vi "WHD_VEten_0.1.3._WS_BIDIR_Calibr.vi"() -> ()   [LabVIEW 2015]
uses:
  <vilib>/LabVIEW Targets/FPGA/cRIO/shared/nicrio_ModuleControls/nicrio_cRIO-9234_DataRatesRing2.ctl
  <vilib>/RTwatchdog.llb/Watchdog expiration actions.ctl
  <vilib>/userDefined/High Color/nirio_resource_hc.ctl
  <vilib>/FPGAPlugInAG/cRIO-9031/niLvFpga_Open_cRIO-9031.vi
  <vilib>/Utility/error.llb/Error Cluster From Error Code.vi
  <vilib>/rvi/errors/niLvFpgaAdjustHostInterfaceError.vi
  <vilib>/Utility/file.llb/Write Delimited Spreadsheet (string).vi
  <vilib>/FPGAPlugInAG/cRIO-9031/niLvFpga_Run_cRIO-9031.vi
  <vilib>/rvi/interface/common/niFpgaWaitOnOcc.vi
  <vilib>/FPGAPlugInAG/cRIO-9031/niLvFpga_Reset_cRIO-9031.vi
  <vilib>/Utility/config.llb/Write Key (Double).vi
  <vilib>/FPGAPlugInAG/cRIO-9031/niLvFpga_Close_cRIO-9031.vi
  <vilib>/rvi/interface/nirviOpenFPGA/nirviOpenFPGA.xnode
  FPGA Bitfiles/W&RDArabia_FPGATarget_FPGA8a2wsBIdirec_yJvL9yuTbZw.lvbitx
  <vilib>/rvi/interface/nirviReadWriteControl/nirviReadWriteControl.xnode
  <vilib>/rvi/interface/nirviMethod/nirviMethod.xnode
  <vilib>/rvi/interface/nirviCloseFPGA/nirviCloseFPGA.xnode
  <vilib>/NI_Real-Time Target Support.lvlib
  <vilib>/rvi/errors/niLvFpgaMergeErrorWithErrorCode.vi
  AURA_Wheel/Json2Labv.lvlib
  AURA_Wheel/AuraWheelAPI/AuraWheel.lvlib
  NiFpgaLv.dll
  <vilib>/FPGAPlugInAG/cRIO-9031/niLvFpga_ConfigureFifo_cRIO-9031.vi
  <vilib>/FPGAPlugInAG/cRIO-9031/niLvFpga_StartFifo_cRIO-9031.vi
  <vilib>/FPGAPlugInAG/cRIO-9031/niLvFpga_ReadFifo_cRIO-9031.vi
  <vilib>/FPGAPlugInAG/cRIO-9031/niLvFpga_StopFifo_cRIO-9031.vi
  <vilib>/Utility/config.llb/NI_LVConfig.lvlib
panel:
  in  "Developer commad":string
  out "Save calibration":bool
  out "calibration log":path
  out "Pattern amplitude (g)":dbl=1.02
  out "Pattern frequency (Hz)":dbl=159.2
  out "Folder":path
  out "Report":string
  out "path calib":path
  out "AURA wheel test":bool
  out "LOG.txt":path
  out "Report_AURA":string
  out "RFID_Error":errorcluster
  out "error FPGA":errorcluster
  out "error AURA":errorcluster
  out "error manipulacion archivos":errorcluster
  out "Response headers":string
  out "Max RMS Ruedas":dbl[][](array[numeric])
  out "TAGs LR6":string[](array[string])
  out "TAGs HEX":string[](array[string])
  out "Parar":bool
  out "result":bool
  out "TAGs":string[](array[string])
  out "Temperatura (ºC)":dbl
  out "V (m/s)":dbl
  out "Digital?":bool=TRUE
  out "Watchdog config":T1={"reset"=FALSE, "occurrence"=FALSE, "trigger protocol"=enum."active high", "trigger line"=enum."none", "disable watchdog on VI exit"=TRUE}
  out "Tiempo de adquisicion":dbl=10.0
  out "Adquirir":bool
  out "Nº Ruedas 1":i32
  out "NºRuedas 2":i32
  out "Disco Duro Disponible (bytes)":i64
  out "Buffer Overflow":bool
  out "Buffer Underflow":bool
  out "Archivo\nvalido?":bool
  out "Número de ejes detectados":i32
  out "Ejes_convoy":i32
  out "Tiempo de paso (s)":dbl
  out "created path":path
  out "Nombre de archivo":path[](array[path])
  out "LR6 IP address":string="192.168.106.94"
  out "Port LR6":u16=2001
  out "T fuera rango":bool
  out "Frecuencia de muestreo (Hz)":dbl=25600.0
  out "Escaneos de la FIFO por canal":u32=5000
  out "Tiempo extra al detector de paso (s)":dbl=1.0
  out "dt RMS":dbl=256.0
  out "Frecuencia de muestreo y módulo CRIO":T2=2 items=["51.200 kS/s (NI 9234)"=1, "25.600 kS/s (NI 9234)"=2, "17.067 kS/s (NI 9234)"=3, "12.800 kS/s (NI 9234)"=4, "10.240 kS/s (NI 9234)"=5, "8.533 kS/s (NI 9234)"=6, "7.314 kS/s (NI 9234)"=7, "6.400 kS/s (NI 9234)"=8, "5.689 kS/s (NI 9234)"=9, "5.120 kS/s (NI 9234)"=10, "4.654 kS/s (NI 9234)"=11, "4.267 kS/s (NI 9234)"=12, "3.938 kS/s (NI 9234)"=13, "3.657 kS/s (NI 9234)"=14, "3.413 kS/s (NI 9234)"=15, "3.200 kS/s (NI 9234)"=16, "3.012 kS/s (NI 9234)"=17, "2.845 kS/s (NI 9234)"=18, "2.695 kS/s (NI 9234)"=19, "2.560 kS/s (NI 9234)"=20, "2.438 kS/s (NI 9234)"=21, "2.328 kS/s (NI 9234)"=22, "2.226 kS/s (NI 9234)"=23, "2.133 kS/s (NI 9234)"=24, "2.048 kS/s (NI 9234)"=25, "1.969 kS/s (NI 9234)"=26, "1.896 kS/s (NI 9234)"=27, "1.829 kS/s (NI 9234)"=28, "1.765 kS/s (NI 9234)"=29, "1.707 kS/s (NI 9234)"=30, "1.652 kS/s (NI 9234)"=31]
  out "Puerto RFID":u16=2189
  out "IP RFID":string="192.168.106.99"
  out "Offset_rueda WS 2":fxp<+/-,24,-4>=0.004999998956918716 format="%.27g"
  out "Count(mSec)":u32=2
  out "RFID NEM on?":bool
  out "RFID LR6 on?":bool
  out "Canal cero WS1?":bool
  out "Canal cero WS2":bool
  out "Inicio pasada 2":timestamp
  in  "Calibration":bool
  out "Direccion 0?":bool
  out "Boton Adquirir?":bool
  out "RuedaDetectada2?":bool=TRUE
  out "RuedaDetectada1?":bool=TRUE
  out "Timeout ruedas":dbl
  out "Borrar archivos\nadquisicion con error":bool
  out "Able watchdog?":bool
  out "Reset watchdog?":bool
  out "Leer config RFID NEM":bool
  out "bytes to read":i32
  out "DeviceAddress":u8
  out "timeout ms (60000)":i32
  out "Max archivos":u32=2
  out "Bytes libre despues de borrar":u32=2
  out "Bytes min libre":u32=2
  out "Nº de acelerómetros":i32
  out "Nº inductivos":i32
  out "Offset_rueda WS 1":fxp<+/-,24,-4>=0.004999998956918716 format="%.27g"
  out "TAGs_AURAwheel":string[][](array[string])
  out "Plataformas?":bool
  out "Nº Ejes":i32[](array[numeric])
  out "Nº UTs":i32
  out "it-read-LR6":i32[](array[numeric])
  out "it-LR6":i32
  out "RFID_LR6_Error":errorcluster
  out "Series_flota":string[](array[string])
  out "Tabla_flota":string[][](array[string])
  out "Puntos medios de las ventanas":dbl[][](array[numeric])
  out "configuration file path":path=path "c:/Parametros.cfg"
  out "IP synchr":string
  out "data":cluster{"status":string}
  out "confRFID":path=path "c:/RFID/TAGS.csv"
  out "TAGS leidos":path=path "c:/RFID/TAGS.csv"
  out "Use Aura?":bool
  out "Parametros AuraWheel":string[](array[string])
  out "Parámetros acelerómetros":dbl[](array[numeric])
  out "Fin":bool
  out "Contador":i32=1
  out "Path LOG":path=path "c:/TEST"
  out "Fallo fotocelula":bool
  out "Path_Borrar":path=path "c:/Trenes"
  out "Longitud de la unidad":dbl
  out "Aviso no detección":string
  out "Time to Acquire Block (ms)":i32
  out "Distancia de acelerómetros":dbl[](array[numeric])
  out "Block Size":u32
  out "Distancias generales":dbl[](array[numeric])
  out "Reset del controlador":bool
  out "Parar la aplicación":bool
  out "date/time string":string
  out "Timeout ruedas":bool
  out "Tiempo":dbl
  out "Inicio pasada":timestamp
  out "Ultimo TEST":timestamp
  out "Fuente":bool=TRUE
  out "RFID_ID":refnum<k5>
  out "DC OK":string
  out "Aviso temperatura":string
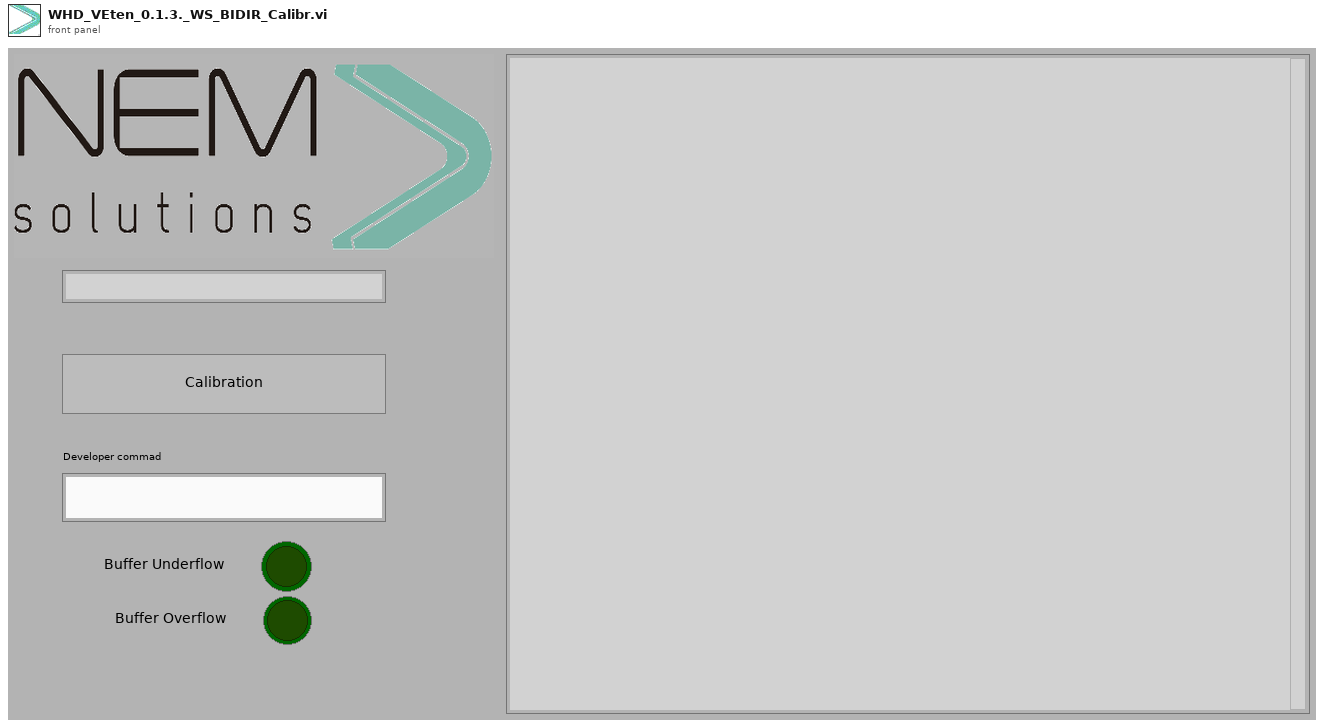
[diagram p1: front panel]
types:
  T1 = typedef "Watchdog expiration actions.ctl" = cluster{"reset":bool, "occurrence":bool, "trigger protocol":enum16{"active high", "active low", "open collector"}, "trigger line":enum16{"none", "line 0", "line 1", "line 2", "line 3", "line 4", "line 5", "line 6", "line 7", "SMB line 0"}, "disable watchdog on VI exit":bool}
  T2 = typedef "nicrio_cRIO-9234_DataRatesRing2.ctl" = u8
  T3 = typedef "nirio_resource_hc.ctl" = tag
  T4 = enum16{"Standard", "Buffered", "CRLF", "Immediate"}
  T5 = enum16{"open", "replace", "create", "open or create", "replace or create", "replace or create with confirmation"}
  T6 = enum16{"big-endian, network order", "native, host order", "little-endian"}
  T7 = cluster{"error IO":errorcluster, bool[], u32[], string[], dbl[]}
  T8 = cluster{"error out":errorcluster, dbl[], "TAGs":string[], "Direccion 0?":bool}
  T9 = cluster{"g_ts":dbl, "p_sp":dbl, "p_tp":dbl, "p_tg":cluster{"tg_n":dbl, "tg_t":string}[], "p_ax":cluster{"ax_n":dbl, "ax_sp":dbl, "ax_wh":cluster{"wh_p":dbl, "wh_a1":dbl, "wh_a2":dbl, "wh_a3":dbl, "wh_a4":dbl}[]}[]}
  T10 = cluster{"Frecuencia de muestreo y módulo CRIO":T2, "Count(mSec)":u32, "Frecuencia de muestreo (Hz)":dbl, "Escaneos de la FIFO por canal":u32, "Nº inductivos":i32, "Nº de acelerómetros":i32}
  T11 = typedef "NI_LVConfig.lvlib/Config Data RefNum.ctl" = refnum<k1>
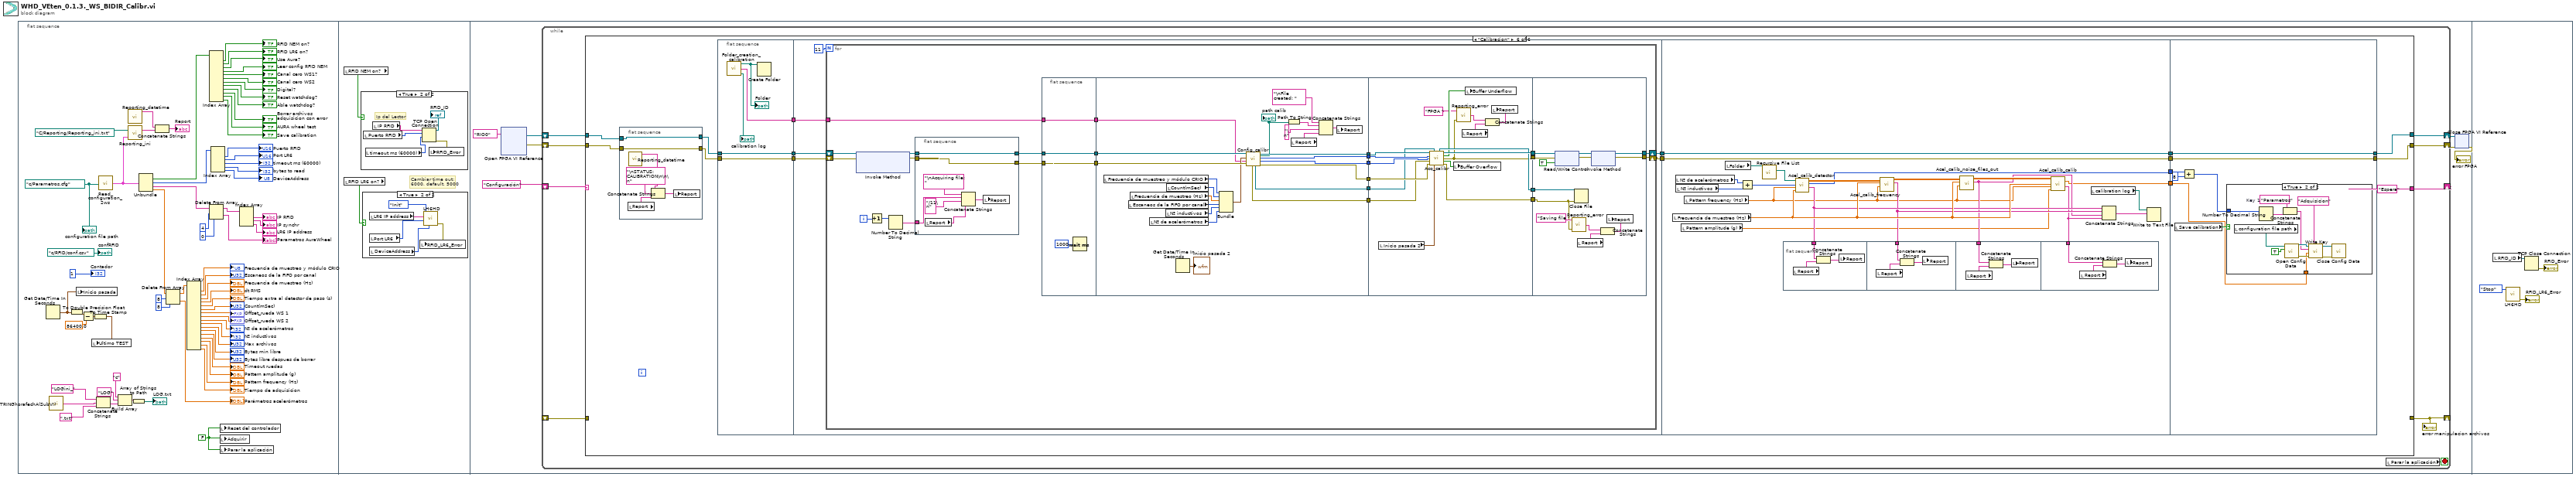
[diagram p0: block diagram]
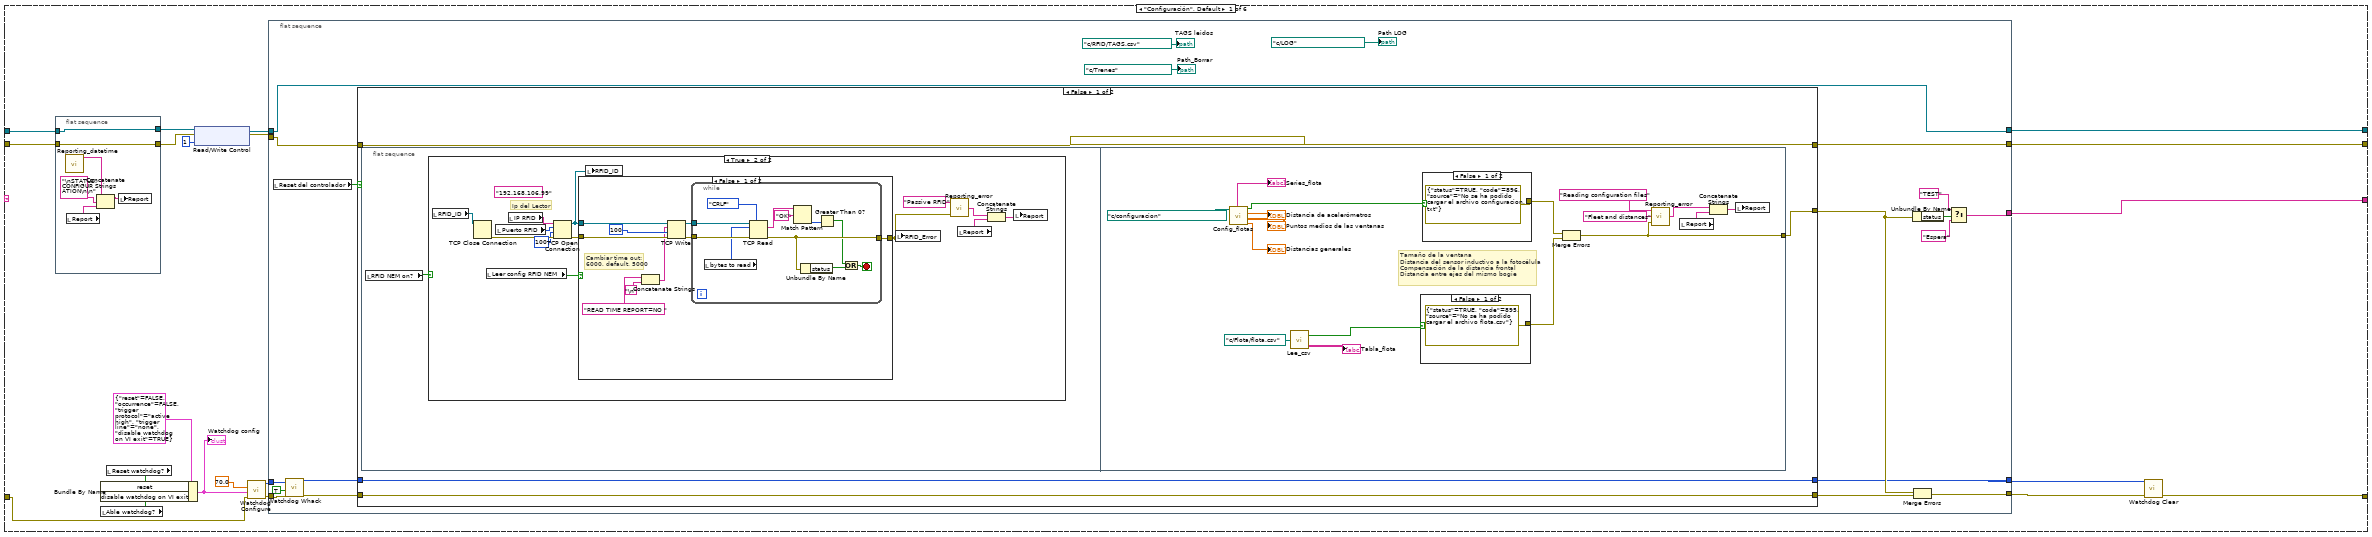
[diagram p4: hidden frame]
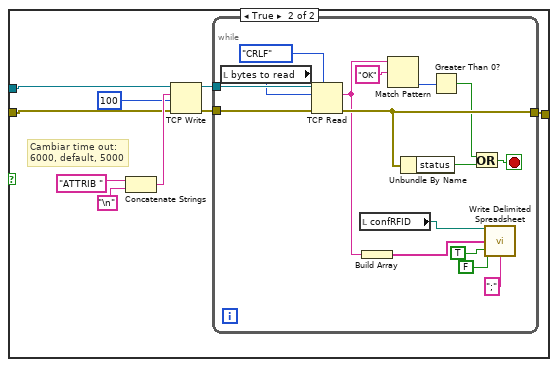
[diagram p6: hidden frame]
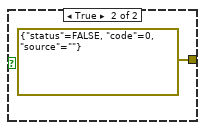
[diagram p7: hidden frame]
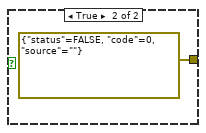
[diagram p8: hidden frame]
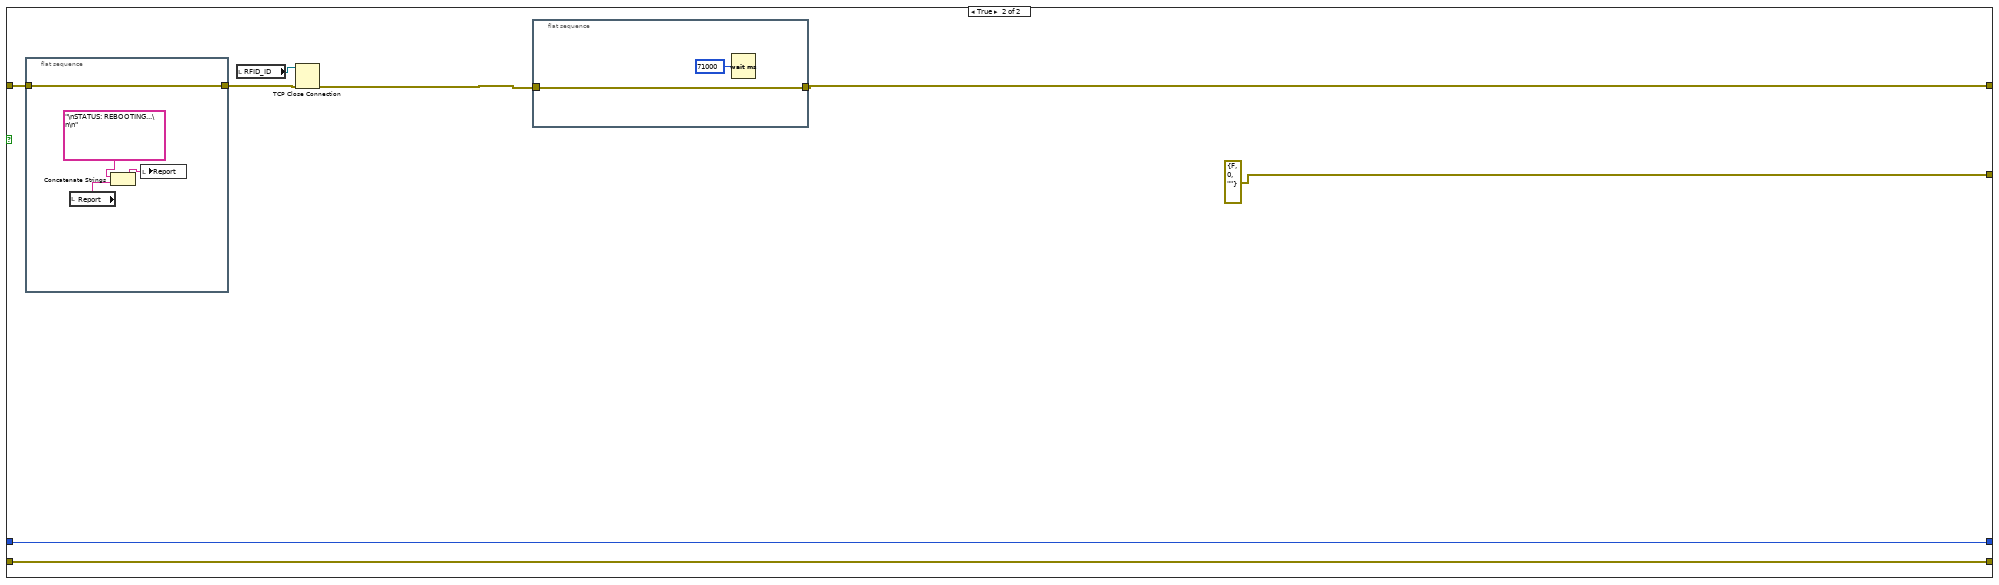
[diagram p9: hidden frame]
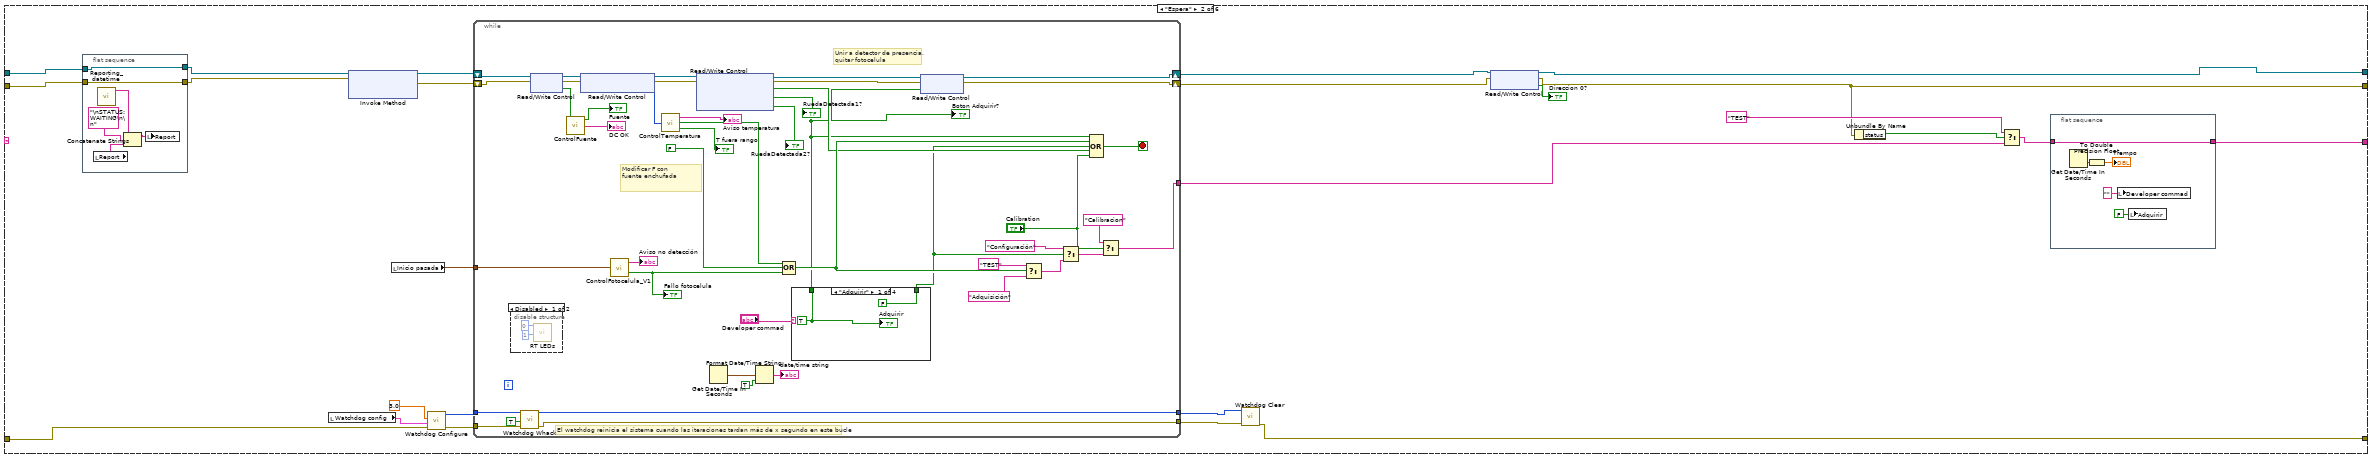
[diagram p10: hidden frame]
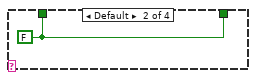
[diagram p11: hidden frame]
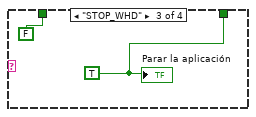
[diagram p12: hidden frame]
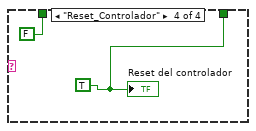
[diagram p13: hidden frame]
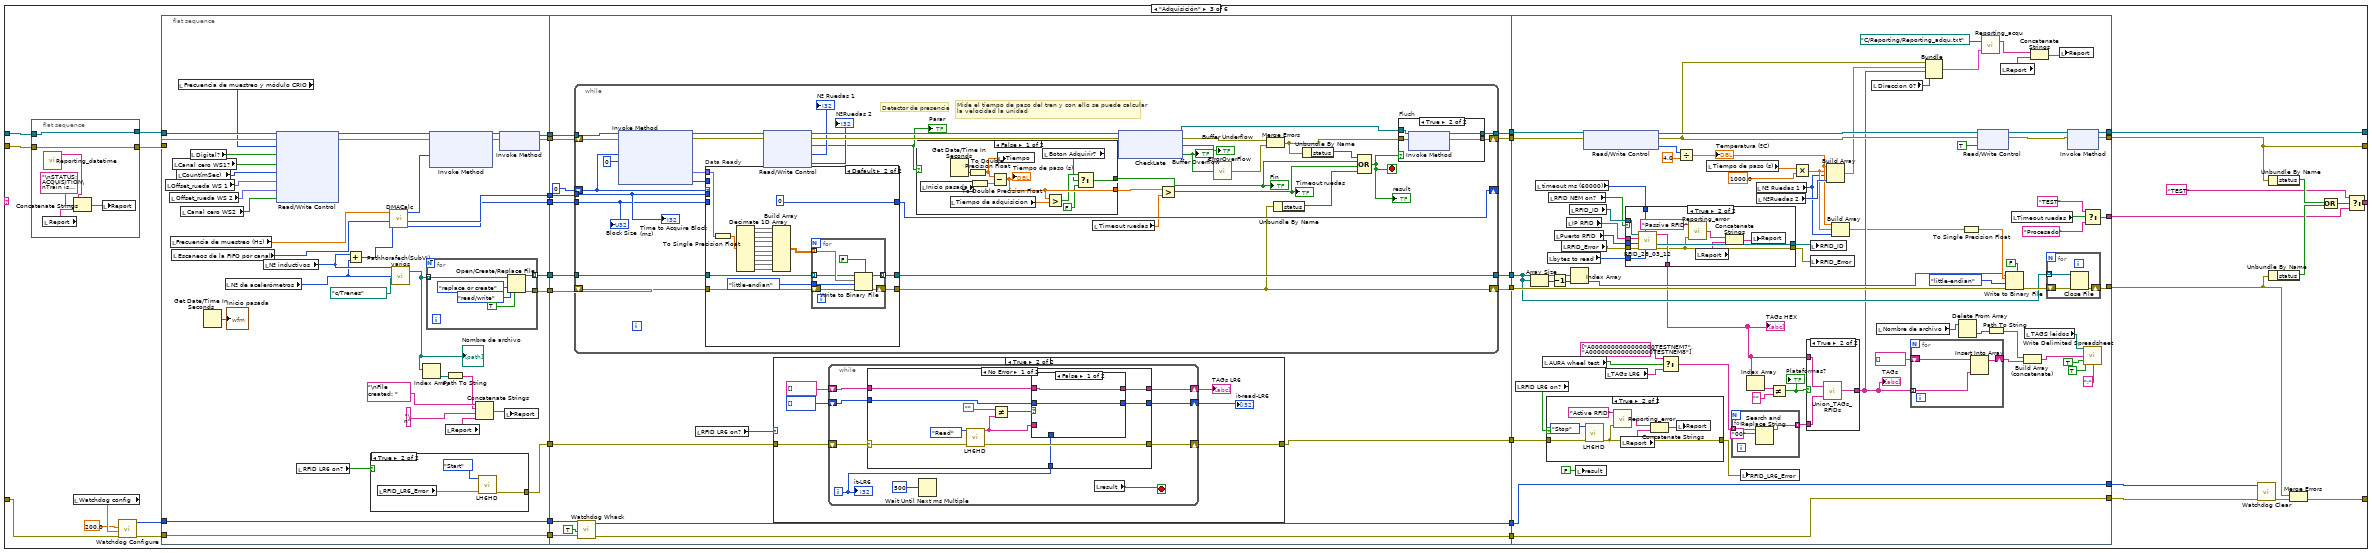
[diagram p15: hidden frame]
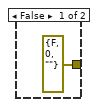
[diagram p16: hidden frame]
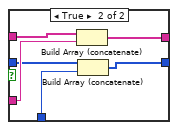
[diagram p18: hidden frame]
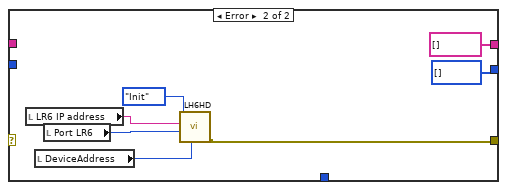
[diagram p19: hidden frame]
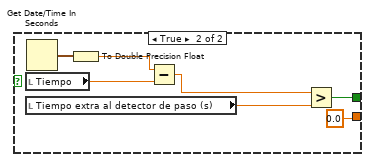
[diagram p20: hidden frame]
diagram:
  n1 = flat-sequence {
    frame #0 {
      w1 = FALSE ("Reset del controlador")
      w63 = path "c:/Parametros.cfg" ("configuration file path")
      n2 = Get Date/Time In Seconds() -> (seconds since 1Jan1904=w68:timestamp)
      n3 = call "STRINGhorafechA(SubVI).vi"() -> ("STRINGhora_fecha"=w12:string)
      n4 = To Double Precision Float(number=w68) -> (double precision float=w70:dbl)
      n5 = local write "Inicio pasada"(w68) -> ()
      n6 = Subtract(x=w70, y=86400.0) -> (x-y=w69:dbl)
      n7 = To Time Stamp(1:w69) -> (0:w67:timestamp)
      n8 = local write "Ultimo TEST"(w67) -> ()
      n9 = Concatenate Strings("LOGini_" ("string"), w12, ".txt" ("string")) -> (w14:string)
      n10 = call "Read_configuration_2ws.vi"("configuration file path"=w63) -> ("output cluster"=w18:T7)
      n11 = Build Array("c", "LOG" ("element"), w14) -> (w11:string[])
      n12 = call "Reporting_ini.vi"("Configuration cluster"=w18, "address repoting"=path "C:/Reporting/Reporting_ini.txt" ("file (use dialog)")) -> ("Reporting"=w17:string)  [unwired: 1 in]
      n13 = call "Reporting_datetime.vi"() -> ("String"=w15:string)  [unwired: 11 in]
      n14 = Array of Strings to Path(0:w11) -> (2:→"LOG.txt":path)  [unwired: 1 out]
      n15 = Unbundle(w18) -> (w66:bool[], w65:u32[], w58:string[], w62:dbl[])  [unwired: 1 out]
      n16 = Concatenate Strings(w15, w17) -> (→"Report":string)
      n17 = Delete From Array(array=w62, length=8, index=8) -> (deleted portion=→"Parámetros acelerómetros":dbl[], array with subset deleted=w61:dbl[])
      n18 = Index Array(array=w61) -> (element #1=→"Frecuencia de muestreo y módulo CRIO":dbl, element #2=→"Escaneos de la FIFO por canal":dbl, element #3=→"Frecuencia de muestreo (Hz)":dbl, element #4=→"dt RMS":dbl, element #5=→"Tiempo extra al detector de paso (s)":dbl, element #6=→"Count(mSec)":dbl, element #7=→"Offset_rueda WS 1":dbl, element #8=→"Offset_rueda WS 2":dbl, element #9=→"Nº de acelerómetros":dbl, element #10=→"Nº inductivos":dbl, element #11=→"Max archivos":dbl, element #12=→"Bytes min libre":dbl, element #13=→"Bytes libre despues de borrar":dbl, element #14=→"Timeout ruedas":dbl, element #15=→"Pattern amplitude (g)":dbl, element #16=→"Pattern frequency (Hz)":dbl, element #17=→"Tiempo de adquisicion":dbl)  [unwired: 17 in]
      n19 = Index Array(array=w66) -> (element #1=→"RFID NEM on?":bool, element #2=→"RFID LR6 on?":bool, element #3=→"Use Aura?":bool, element #4=→"Leer config RFID NEM":bool, element #5=→"Canal cero WS1?":bool, element #6=→"Canal cero WS2":bool, element #7=→"Digital?":bool, element #8=→"Reset watchdog?":bool, element #9=→"Able watchdog?":bool, element #10=→"Borrar archivos\nadquisicion con error":bool, element #11=→"AURA wheel test":bool, element #12=→"Save calibration":bool)  [unwired: 12 in]
      n20 = Delete From Array(array=w58, length=4, index=0) -> (deleted portion=→"Parametros AuraWheel":string[], array with subset deleted=w57:string[])
      n21 = Index Array(array=w65) -> (element #1=→"Puerto RFID":u32, element #2=→"Port LR6":u32, element #3=→"timeout ms (60000)":u32, element #4=→"bytes to read":u32, element #5=→"DeviceAddress":u32)  [unwired: 5 in]
      n22 = local write "Reset del controlador"(w1) -> ()
      n23 = local write "Adquirir"(w1) -> ()
      n24 = local write "Parar la aplicación"(w1) -> ()
      n25 = Index Array(array=w57) -> (element #1=→"IP RFID":string, element #2=→"IP synchr":string, element #3=→"LR6 IP address":string)  [unwired: 3 in]
      "Contador" <- 1
      "confRFID" <- path "c:/RFID/conf.csv" ("file path (use dialog)")
      "configuration file path" <- w63
    }
    frame #1 {
      # "Cambiar time out:\n6000, default, 5000"
      n26 = local read "RFID NEM on?"() -> (w73:bool)
      n27 = local read "RFID LR6 on?"() -> (w72:bool)
      n28 = case shown="True" w73 {
        frame False {
        }
        frame True {
          # "Ip del Lector"
          n29 = local read "Puerto RFID"() -> (w81:u16)
          n30 = local read "timeout ms (60000)"() -> (w79:i32)
          n31 = local read "IP RFID"() -> (w82:string)
          n32 = TCP Open Connection(address=w82, remote port or service name=w81, timeout ms (60000)=w79) -> (connection ID=→"RFID_ID":refnum<k5>, error out=w80:errorcluster)  [unwired: 1 in, 1 out]
          n33 = local write "RFID_Error"(w80) -> ()
        }
      }
      n34 = case shown="True" w72 {
        frame False {
        }
        frame True {
          n35 = local read "LR6 IP address"() -> (w74:string)
          n36 = local read "Port LR6"() -> (w75:u16)
          n37 = local read "DeviceAddress"() -> (w76:u8)
          n38 = call "LH6HD.vi"("DeviceAddress"=w76, "Reader Port"=w75, "IP Address"=w74, "Action"=enum16{"Init", "Start", "Read", "Stop", "Exit"}."Init") -> ("error out"=w78:errorcluster)  [unwired: 6 in, 1 out]
          n39 = local write "RFID_LR6_Error"(w78) -> ()
        }
      }
    }
    frame #2 {
      n40 = xnode "Open FPGA VI Reference"("resource name"=T3 "RIO0") -> ("FPGA VI Reference Out"=w90:refnum<k20>, "error out"=w89:errorcluster)  [unwired: 1 in]
      n41 = while {
        shift-right: [w91] -> _
        shift-left: "Configuración" -> [w99]
        shift-right: [w93] -> w86
        shift-left: w90 -> [w98]
        shift-right: [w92] -> w85
        shift-left: w89 -> [w97]
        shift-right: [w96] -> _
        shift-left: _ -> [w95]
        stop <- w94 stop-if-true
        n42 = case shown="\"Calibracion\"" w99 {
          tunnel: [w109 w262 w352 w709 w957 "Espera"] -> w91
          tunnel: [w119 w250 w366 w698 w956 w1030] -> w93
          tunnel: [w120 w249 w367 w696 w955 w1029] -> w92
          tunnel: w98 -> [w103 w248 w338 w699 w956 w1035]
          tunnel: w97 -> [w102 w247 w337 w697 w948 w1034]
          tunnel: [w116 w256 w364 w694 w947 _] -> w96
          tunnel: w95 -> [w108 w261 w348 w708 w944 _]
          frame "Configuración", Default {
            n43 = flat-sequence {
              tunnel: w103 -> [w126]
              tunnel: w102 -> [w125]
              tunnel: [w126] -> w101
              tunnel: [w125] -> w100
              frame #0 {
                n44 = call "Reporting_datetime.vi"() -> ("String"=w121:string)  [unwired: 11 in]
                n45 = local read "Report"() -> (w122:string)
                n46 = Concatenate Strings(w121, "\nSTATUS: CONFIGURATION\n\n", w122) -> (w124:string)
                n47 = local write "Report"(w124) -> ()
              }
            }
            n48 = local read "Able watchdog?"() -> (w113:bool)
            n49 = local read "Reset watchdog?"() -> (w114:bool)
            n50 = Bundle By Name(cluster=T1 {"reset"=FALSE, "occurrence"=FALSE, "trigger protocol"=enum."active high", "trigger line"=enum."none", "disable watchdog on VI exit"=TRUE} ("expiration actions"), "reset"=w114, "disable watchdog on VI exit"=w113) -> (w107:T1)
            "Watchdog config" <- w107
            n51 = xnode "Read/Write Control"("FPGA VI Reference In"=w101, "error in"=w100, "Cycles to Filter"=u16 1) -> ("FPGA VI Reference Out"=w112:refnum<k20>, "error out"=w111:errorcluster)
            n52 = call <vilib>:"Watchdog Configure.vi"("error in (no error)"=w108, "expiration actions"=w107, "timeout (1 sec)"=70.0) -> ("error out"=w104:errorcluster, "watchdogID"=w105:u64)  [unwired: 1 in, 2 out]
            n53 = flat-sequence {
              tunnel: [w137] -> w120
              tunnel: [w145] -> w109
              tunnel: w112 -> [w138]
              tunnel: [w138] -> w119
              tunnel: [w140] -> w117
              tunnel: w111 -> [w135]
              tunnel: [w132] -> w118
              tunnel: w105 -> [w128]
              tunnel: w104 -> [w127]
              frame #0 {
                n54 = local read "Reset del controlador"() -> (w134:bool)
                n55 = call <vilib>:"Watchdog Whack.vi"("error in (no error)"=w127, "reset watchdog after expire? (F)"=TRUE, "watchdogID in"=w128) -> ("error out"=w130:errorcluster, "watchdogID out"=w131:u64)  [unwired: 2 in, 1 out]
                n56 = case shown="False" w134 {
                  tunnel: w135 -> [w150 w233]
                  tunnel: [w150 w236] -> w137
                  tunnel: [w147 errorcluster {"status"=FALSE, "code"=0, "source"=""} ("error IO")] -> w136
                  tunnel: [w149 w235] -> w132
                  tunnel: w131 -> [w149 w235]
                  tunnel: w130 -> [w148 w234]
                  tunnel: [w148 w234] -> w129
                  frame False {
                    n57 = flat-sequence {
                      tunnel: [w210] -> w147
                      frame #0 {
                        n58 = local read "RFID NEM on?"() -> (w151:bool)
                        n59 = case shown="True" w151 {
                          frame False {
                          }
                          frame True {
                            (unwired) "192.168.106.99" ("address")
                            # "Ip del Lector"
                            n60 = local read "RFID_ID"() -> (w163:refnum<k5>)
                            n61 = TCP Close Connection(connection ID=w163) -> (error out=w164:errorcluster)  [unwired: 2 in, 1 out]
                            n62 = local read "Leer config RFID NEM"() -> (w157:bool)
                            n63 = local read "Puerto RFID"() -> (w161:u16)
                            n64 = local read "IP RFID"() -> (w160:string)
                            n65 = TCP Open Connection(address=w160, remote port or service name=w161, timeout ms (60000)=100, error in (no error)=w164) -> (connection ID=w162:refnum<k5>, error out=w158:errorcluster)  [unwired: 1 out]
                            n66 = case shown="False" w157 {
                              tunnel: w162 -> [w173 w187]
                              tunnel: [w171 w185] -> w156
                              tunnel: w158 -> [w168 w186]
                              frame False {
                                # "Cambiar time out:\n6000, default, 5000"
                                n67 = Concatenate Strings("READ TIME REPORT=NO " ("data in"), "\n") -> (w165:string)
                                n68 = TCP Write(connection ID=w173, data in=w165, error in (no error)=w168, 9:100 ("timeout ms (25000)")) -> (connection ID out=w169:refnum<k5>, error out=w170:errorcluster)  [unwired: 1 out]
                                n69 = while {
                                tunnel: w170 -> [w183]
                                tunnel: w169 -> [w182]
                                tunnel: [w181] -> w171
                                stop <- w178 stop-if-true
                                n70 = local read "bytes to read"() -> (w174:i32)
                                n71 = TCP Read(connection ID=w182, bytes to read=w174, error in (no error)=w183, 7:T4."CRLF" ("mode (standard)")) -> (data out=w176:string, error out=w181:errorcluster)  [unwired: 1 in, 1 out]
                                n72 = Match Pattern(string=w176, regular expression="OK") -> (offset past match=w179:i32)  [unwired: 4 out]
                                n73 = Unbundle By Name(w181) -> ("status"=w177:bool)
                                n74 = Greater Than 0?(x=w179) -> (x > 0?=w175:bool)
                                n75 = Or(x=w175, y=w177) -> (x .or. y?=w178:bool)
                                }
                              }
                              frame True {
                                # "Cambiar time out:\n6000, default, 5000"
                                n76 = Concatenate Strings("ATTRIB " ("data in"), "\n") -> (w193:string)
                                n77 = TCP Write(connection ID=w187, data in=w193, error in (no error)=w186, 9:100 ("timeout ms (25000)")) -> (connection ID out=w190:refnum<k5>, error out=w189:errorcluster)  [unwired: 1 out]
                                n78 = while {
                                tunnel: w189 -> [w208]
                                tunnel: w190 -> [w207]
                                tunnel: [w206] -> w185
                                stop <- w203 stop-if-true
                                n79 = local read "bytes to read"() -> (w194:i32)
                                n80 = TCP Read(connection ID=w207, bytes to read=w194, error in (no error)=w208, 7:T4."CRLF" ("mode (standard)")) -> (data out=w197:string, error out=w206:errorcluster)  [unwired: 1 in, 1 out]
                                n81 = local read "confRFID"() -> (w196:path)
                                n82 = Build Array(w197) -> (w195:string[])
                                n83 = Match Pattern(string=w197, regular expression="OK") -> (offset past match=w204:i32)  [unwired: 4 out]
                                n84 = Unbundle By Name(w206) -> ("status"=w202:bool)
                                n85 = Greater Than 0?(x=w204) -> (x > 0?=w201:bool)
                                n86 = Or(x=w201, y=w202) -> (x .or. y?=w203:bool)
                                n87 = call-poly <vilib>:"Write Delimited Spreadsheet.vi"("file path (dialog if empty)"=w196, "1D data"=w195, "append to file? (F)"=FALSE ("transpose? (no:F)"), "transpose? (F)"=TRUE ("append to file? (new file:F)"), "delimiter (\\t)"=";" ("delimiter (\\t)")) -> ()  [unwired: 9 in, 2 out]
                                }
                              }
                            }
                            n88 = local write "RFID_ID"(w162) -> ()
                            n89 = local write "RFID_Error"(w156) -> ()
                            n90 = call "Reporting_error.vi"("error out 2"=w156, "Concept"="Passive RFID") -> ("Reporting"=w153:string)  [unwired: 1 in]
                            n91 = local read "Report"() -> (w154:string)
                            n92 = Concatenate Strings(w153, w154) -> (w152:string)
                            n93 = local write "Report"(w152) -> ()
                          }
                        }
                      }
                      frame #1 {
                        # "Tamaño de la ventana\nDistancia del sensor inductivo a la fotocélula\nCompensación de la distancia frontal\nDistancia entre ejes del mismo bogie"
                        n94 = call "Config_flotas.vi"("file path (dialog if empty)"=path "c:/configuracion") -> ("Distancias generales"=→"Distancias generales":dbl[], "Puntos medios de las ventanas"=→"Puntos medios de las ventanas":dbl[][], "Distancia de acelerómetros"=→"Distancia de acelerómetros":dbl[], "Distacias y medidas de dispositivos"=w223:bool, "Series_flota"=→"Series_flota":string[])  [unwired: 3 in]
                        n95 = call "Lee_csv.vi"("Path"=path "c:/Flota/flota.csv") -> ("Tabla_flota"=→"Tabla_flota":string[][], "Lectura_OK?"=w220:bool)
                        n96 = case shown="False" w220 {
                          tunnel: [errorcluster {"status"=TRUE, "code"=895, "source"="No se ha podido cargar el archivo flota.csv"} ("error out") errorcluster {"status"=FALSE, "code"=0, "source"=""} ("error out")] -> w224
                          frame False {
                          }
                          frame True {
                          }
                        }
                        n97 = case shown="False" w223 {
                          tunnel: [errorcluster {"status"=TRUE, "code"=896, "source"="No se ha podido cargar el archivo configuracion.txt"} ("error out") errorcluster {"status"=FALSE, "code"=0, "source"=""} ("error out")] -> w225
                          frame False {
                          }
                          frame True {
                          }
                        }
                        n98 = Merge Errors(w225, w224) -> (w210:errorcluster)
                        n99 = call "Reporting_error.vi"("error out 2"=w210, "Concept explanation"="Fleet and distances", "Concept"="Reading configuration files") -> ("Reporting"=w212:string)
                        n100 = local read "Report"() -> (w211:string)
                        n101 = Concatenate Strings(w212, w211) -> (w213:string)
                        n102 = local write "Report"(w213) -> ()
                      }
                    }
                  }
                  frame True {
                    n103 = flat-sequence {
                      tunnel: w233 -> [w242]
                      tunnel: [w242] -> w232
                      frame #0 {
                        n104 = local read "Report"() -> (w241:string)
                        n105 = Concatenate Strings("\nSTATUS: REBOOTING...\n\n", w241) -> (w239:string)
                        n106 = local write "Report"(w239) -> ()
                      }
                    }
                    n107 = local read "RFID_ID"() -> (w238:refnum<k5>)
                    n108 = TCP Close Connection(connection ID=w238, error in (no error)=w232) -> (error out=w231:errorcluster)  [unwired: 2 out]
                    n109 = flat-sequence {
                      tunnel: [w244] -> w236
                      tunnel: w231 -> [w244]
                      frame #0 {
                        n110 = Wait (ms)(milliseconds to wait=u32 71000) -> ()  [unwired: 1 out]
                      }
                    }
                  }
                }
                n111 = Unbundle By Name(w136) -> ("status"=w146:bool)
                n112 = Merge Errors(w136, w129) -> (w140:errorcluster)
                n113 = Select(t="TEST", s=w146, f="Espera") -> (s? t:f=w145:string)
                "Path_Borrar" <- path "c:/Trenes" ("file path (use dialog)")
                "Path LOG" <- path "c:/LOG" ("file path (use dialog)")
                "TAGS leidos" <- path "c:/RFID/TAGS.csv" ("file path (use dialog)")
              }
            }
            n114 = call <vilib>:"Watchdog Clear.vi"("error in (no error)"=w117, "watchdogID in"=w118) -> ("error out"=w116:errorcluster)  [unwired: 5 in]
          }
          frame "Espera" {
            n115 = flat-sequence {
              tunnel: w248 -> [w275]
              tunnel: w247 -> [w274]
              tunnel: [w275] -> w246
              tunnel: [w274] -> w245
              frame #0 {
                n116 = local read "Report"() -> (w271:string)
                n117 = call "Reporting_datetime.vi"() -> ("String"=w270:string)  [unwired: 11 in]
                n118 = Concatenate Strings(w270, "\nSTATUS: WAITING\n\n", w271) -> (w273:string)
                n119 = local write "Report"(w273) -> ()
              }
            }
            n120 = local read "Watchdog config"() -> (w255:T1)
            n121 = xnode "Invoke Method"("FPGA VI Reference In"=w246, "error in"=w245) -> ("FPGA VI Reference Out"=w265:refnum<k20>, "error out"=w264:errorcluster)  [unwired: 1 in]
            n122 = local read "Inicio pasada"() -> (w269:timestamp)
            n123 = call <vilib>:"Watchdog Configure.vi"("error in (no error)"=w261, "expiration actions"=w255, "timeout (1 sec)"=3.0) -> ("error out"=w260:errorcluster, "watchdogID"=w259:u64)  [unwired: 1 in, 2 out]
            n124 = while {
              tunnel: [w286] -> w268
              shift-right: [w295] -> w251
              shift-left: w265 -> [w305]
              shift-right: [w294] -> w252
              shift-left: w264 -> [w304]
              tunnel: w269 -> [w308]
              tunnel: w260 -> [w292]
              tunnel: w259 -> [w293]
              tunnel: [w291] -> w258
              tunnel: [w290] -> w257
              stop <- w284 stop-if-true
              # "Modificar F con\nfuente enchufada"
              # "Unir a detector de presencia,\nquitar fotocelula"
              # "El watchdog reinicia el sistema cuando las iteraciones tardan más de x segundo en este bucle"
              n125 = disable-structure shown="Disabled" {
                frame Disabled {
                  n126 = call <vilib>:"RT LEDs.vi"("State"=1, "LED Num"=0) -> ()  [unwired: 1 in, 5 out]
                }
                frame Enabled {
                }
              }
              n127 = call <vilib>:"Watchdog Whack.vi"("error in (no error)"=w292, "reset watchdog after expire? (F)"=TRUE, "watchdogID in"=w293) -> ("error out"=w290:errorcluster, "watchdogID out"=w291:u64)  [unwired: 2 in, 1 out]
              n128 = xnode "Read/Write Control"("FPGA VI Reference In"=w305, "error in"=w304) -> ("FPGA VI Reference Out"=w317:refnum<k20>, "error out"=w316:errorcluster, "DC OK"=w321:bool)
              n129 = call "ControlFuente.vi"("DC OK 3"=w321) -> ("DC OK 2"=→"Fuente":bool, "DC OK"=→"DC OK":string)  [unwired: 1 out]
              n130 = xnode "Read/Write Control"("FPGA VI Reference In"=w317, "error in"=w316) -> ("FPGA VI Reference Out"=w312:refnum<k20>, "error out"=w311:errorcluster, "Chassis Temperature"=w319:i16)
              n131 = call "ControlFotocelula_V1.vi"("Tiempo de entrada a espera"=w308) -> ("Aviso no detección"=→"Aviso no detección":string, "Boolean"=w309:bool)
              "Fallo fotocelula" <- w309
              n132 = call "ControlTemperatura.vi"("Chassis Temperature"=w319) -> ("Aviso temperatura"=→"Aviso temperatura":string, "Boolean"=w313:bool, "T fuera rango"=→"T fuera rango":bool)
              n133 = xnode "Read/Write Control"("FPGA VI Reference In"=w312, "error in"=w311) -> ("FPGA VI Reference Out"=w307:refnum<k20>, "error out"=w306:errorcluster, "Detector de presencia"=w300:bool, "RuedaDetectada1?"=→"RuedaDetectada1?":bool, "RuedaDetectada2?"=→"RuedaDetectada2?":bool)
              n134 = Get Date/Time In Seconds() -> (seconds since 1Jan1904=w302:timestamp)
              n135 = Format Date/Time String(seconds (now)=w302, UTC format=TRUE) -> (date/time string=→"date/time string":string)  [unwired: 1 in]
              n136 = Compound Arithmetic op=OR(w313, FALSE ("value"), w309) -> (w310:bool)
              n137 = case shown="\"Adquirir\"" "Developer commad" {
                tunnel: [w327 w328 FALSE ("Adquirir") FALSE ("Adquirir")] -> w283
                tunnel: [FALSE ("Adquirir") w328 w329 w331] -> w282
                frame "Adquirir" {
                  w327 = TRUE ("Adquirir")
                  "Adquirir" <- w327
                }
                frame Default {
                  w328 = FALSE ("Adquirir")
                }
                frame "STOP_WHD" {
                  w329 = TRUE ("Adquirir")
                  "Parar la aplicación" <- w329
                }
                frame "Reset_Controlador" {
                  w331 = TRUE ("Adquirir")
                  "Reset del controlador" <- w331
                }
              }
              "Boton Adquirir?" <- w283
              n138 = xnode "Read/Write Control"("FPGA VI Reference In"=w307, "error in"=w306, "Fotocélula"=w283) -> ("FPGA VI Reference Out"=w295:refnum<k20>, "error out"=w294:errorcluster)
              n139 = Select(t="TEST", s=w310, f="Adquisición") -> (s? t:f=w322:string)
              n140 = Select(t="Configuración", s=w282, f=w322) -> (s? t:f=w288:string)
              n141 = Compound Arithmetic op=OR(w283, w310, w282, w300, "Calibration") -> (w284:bool)
              n142 = Select(t="Calibracion", s="Calibration", f=w288) -> (s? t:f=w286:string)
            }
            n143 = call <vilib>:"Watchdog Clear.vi"("error in (no error)"=w257, "watchdogID in"=w258) -> ("error out"=w256:errorcluster)  [unwired: 5 in]
            n144 = xnode "Read/Write Control"("FPGA VI Reference In"=w251, "error in"=w252) -> ("FPGA VI Reference Out"=w250:refnum<k20>, "error out"=w249:errorcluster, "Direccion 0?"=→"Direccion 0?":bool)
            n145 = Unbundle By Name(w249) -> ("status"=w267:bool)
            n146 = Select(t="TEST", s=w267, f=w268) -> (s? t:f=w263:string)
            n147 = flat-sequence {
              tunnel: [w279] -> w262
              tunnel: w263 -> [w279]
              frame #0 {
                n148 = Get Date/Time In Seconds() -> (seconds since 1Jan1904=w280:timestamp)
                n149 = To Double Precision Float(number=w280) -> (double precision float=→"Tiempo":dbl)
                n150 = local write "Developer commad"("" ("Developer commad")) -> ()
                n151 = local write "Adquirir"(FALSE ("Adquirir")) -> ()
              }
            }
          }
          frame "Adquisición" {
            n152 = flat-sequence {
              tunnel: w338 -> [w378]
              tunnel: w337 -> [w377]
              tunnel: [w378] -> w336
              tunnel: [w377] -> w335
              frame #0 {
                n153 = local read "Report"() -> (w374:string)
                n154 = call "Reporting_datetime.vi"() -> ("String"=w373:string)  [unwired: 11 in]
                n155 = Concatenate Strings(w373, "\nSTATUS: ACQUISITION\nTrain is passing\n\n", w374) -> (w376:string)
                n156 = local write "Report"(w376) -> ()
              }
            }
            n157 = local read "Watchdog config"() -> (w349:T1)
            n158 = call <vilib>:"Watchdog Configure.vi"("error in (no error)"=w348, "expiration actions"=w349, "timeout (1 sec)"=200.0) -> ("error out"=w346:errorcluster, "watchdogID"=w347:u64)  [unwired: 1 in, 2 out]
            n159 = flat-sequence {
              tunnel: w335 -> [w412]
              tunnel: w336 -> [w413]
              tunnel: [w411] -> w363
              tunnel: [w410] -> w362
              tunnel: [w409] -> w361
              tunnel: [w408] -> w360
              tunnel: [w407] -> w359
              tunnel: [w406] -> w358
              tunnel: [w396] -> w351
              tunnel: w347 -> [w395]
              tunnel: w346 -> [w394]
              tunnel: [w395] -> w345
              tunnel: [w394] -> w344
              tunnel: [w428] -> w372
              tunnel: [w445] -> w371
              tunnel: [w444] -> w370
              tunnel: [w443] -> w369
              tunnel: [w436] -> w368
              tunnel: w363 -> [w442]
              tunnel: w362 -> [w441]
              tunnel: w361 -> [w440]
              tunnel: w360 -> [w439]
              tunnel: w359 -> [w438]
              tunnel: w358 -> [w437]
              tunnel: w351 -> [w434]
              tunnel: [w433] -> w350
              tunnel: w345 -> [w432]
              tunnel: w344 -> [w431]
              tunnel: [w429] -> w343
              tunnel: w372 -> [w609]
              tunnel: w371 -> [w604]
              tunnel: w370 -> [w603]
              tunnel: w369 -> [w623]
              tunnel: [w650] -> w355
              tunnel: w368 -> [w652]
              tunnel: [w639] -> w365
              tunnel: [w640] -> w367
              tunnel: [w641] -> w366
              tunnel: w350 -> [w618]
              tunnel: w343 -> [w610]
              tunnel: [w610] -> w341
              tunnel: [w609] -> w340
              frame #0 {
                n160 = local read "Offset_rueda WS 1"() -> (w389:fxp<+/-,24,-4>)
                n161 = local read "Offset_rueda WS 2"() -> (w390:fxp<+/-,24,-4>)
                n162 = local read "Frecuencia de muestreo (Hz)"() -> (w404:dbl)
                n163 = local read "Escaneos de la FIFO por canal"() -> (w393:u32)
                n164 = local read "Canal cero WS1?"() -> (w398:bool)
                n165 = local read "Count(mSec)"() -> (w397:u32)
                n166 = local read "Frecuencia de muestreo y módulo CRIO"() -> (w400:T2)
                n167 = local read "Canal cero WS2"() -> (w388:bool)
                n168 = local read "Digital?"() -> (w399:bool)
                n169 = Get Date/Time In Seconds() -> (seconds since 1Jan1904=→"Inicio pasada":timestamp)
                n170 = local read "Nº de acelerómetros"() -> (w386:i32)
                n171 = local read "Nº inductivos"() -> (w387:i32)
                n172 = xnode "Read/Write Control"("FPGA VI Reference In"=w413, "error in"=w412, "Data Rate"=w400, "Digital?"=w399, "Canal cero WS1?"=w398, "Count(mSec)"=w397, "Offset_WS1"=w389, "Offset_WS2"=w390, "Canal cero WS2?"=w388) -> ("FPGA VI Reference Out"=w403:refnum<k20>, "error out"=w402:errorcluster)
                n173 = local read "RFID LR6 on?"() -> (w391:bool)
                n174 = Add(x=w387, y=w386) -> (x+y=w392:i32)
                n175 = case shown="True" w391 {
                  tunnel: [errorcluster {"status"=FALSE, "code"=0, "source"=""} ("error out") w418] -> w396
                  frame False {
                  }
                  frame True {
                    n176 = local read "RFID_LR6_Error"() -> (w419:errorcluster)
                    n177 = call "LH6HD.vi"("error in (no error)"=w419, "Action"=enum16{"Init", "Start", "Read", "Stop", "Exit"}."Start") -> ("error out"=w418:errorcluster)  [unwired: 8 in, 1 out]
                  }
                }
                n178 = call "DMACalc.vi"("Number of Channels"=w392, "Number of Samples"=w393, "Rate (Hz)"=w404) -> ("Block Size"=w408:u32, "Time to Acquire Block (ms)"=w409:i32, "Host Buffer Size"=w414:u32)  [unwired: 6 in]
                n179 = call "Pathhorafech(SubVI)_varios.vi"("Folder path"=path "c:/Trenes", "Nº de acelerómetros"=w386, "Nº inductivos"=w387) -> ("Acel_Paths"=w382:path[])  [unwired: 1 in, 1 out]
                "Nombre de archivo" <- w382
                n180 = Index Array(array=w382) -> (element=w381:path)  [unwired: 1 in]
                n181 = for {
                  tunnel: w382 -> [w423] mode=indexing
                  tunnel: [w422] -> w407 mode=indexing
                  tunnel: [w421] -> w406
                  n182 = Open/Create/Replace File(file path (use dialog)=w423, operation (0:open)=T5."replace or create", access (0:read/write)=enum16{"read/write", "read-only", "write-only"}."read/write", disable buffering (F)=TRUE) -> (refnum out=w422:refnum<file>, error out=w421:errorcluster)  [unwired: 1 in, 2 out]
                }
                n183 = xnode "Invoke Method"("FPGA VI Reference In"=w403, "error in"=w402, "Requested Depth"=w414) -> ("FPGA VI Reference Out"=w416:refnum<k20>, "error out"=w415:errorcluster)  [unwired: 1 out]
                n184 = local read "Report"() -> (w385:string)
                n185 = Path To String(path=w381) -> (string=w379:string)
                n186 = Concatenate Strings("\nFile created: ", w379, "\n", w385) -> (w384:string)
                n187 = xnode "Invoke Method"("FPGA VI Reference In"=w416, "error in"=w415) -> ("FPGA VI Reference Out"=w411:refnum<k20>, "error out"=w410:errorcluster)
                n188 = local write "Report"(w384) -> ()
              }
              frame #1 {
                n189 = while "Data Acquisition" {
                  tunnel: w442 -> [w496]
                  shift-right: [w520] -> _
                  shift-left: u32 0 ("t") -> [w516]
                  tunnel: w440 -> [w521]
                  tunnel: w439 -> [w519]
                  shift-right: [w522] -> w444
                  shift-left: w441 -> [w513]
                  tunnel: [w517] -> w445
                  tunnel: w438 -> [w500]
                  tunnel: [w501] -> w443
                  shift-right: [w499] -> w436
                  shift-left: w437 -> [w509]
                  stop <- w518 stop-if-true
                  # "Detector de presencia"
                  # "Mide el tiempo de paso del tren y con ello se puede calcular\nla velocidad la unidad"
                  n190 = xnode "Invoke Method"("FPGA VI Reference In"=w496, "error in"=w513, "Number of Elements"=w516, "Timeout (ms)"=0) -> ("FPGA VI Reference Out"=w493:refnum<k20>, "error out"=w498:errorcluster, "Data"=w512:fxp<+/-,24,4>[], "Elements Remaining"=w514:u32)
                  n191 = case "Data Ready" shown="Default" w516 {
                    tunnel: w521 -> [w544 _]
                    tunnel: [w543 u32 0 ("t")] -> w520
                    tunnel: w519 -> [w545 _]
                    tunnel: w514 -> [w542 _]
                    tunnel: w512 -> [_ w567]
                    tunnel: w509 -> [w541 w566]
                    tunnel: [w541 w568] -> w499
                    tunnel: w500 -> [w540 w565]
                    tunnel: [w540 w564] -> w501
                    frame 0 {
                      # "En este caso se compara los elementos que quedan\nen la FIFO del controlador con el tamaño dell bloque\nque aparece en el panel frontal. Si el número de \nelementos en la FIFO es mayor o igual que el tamaño\n del bloque se pasa al siguiente caso y se guardan \nlos datos en un archivo. El reloj que aparece es una\nespera para no consumir recursos."
                      n192 = Greater Or Equal?(x=w542, y=w545) -> (x >= y?=w546:bool)
                      n193 = case shown="False" w546 {
                        tunnel: [u32 0 ("Block Size") w550] -> w543
                        tunnel: [w549 0 ("t")] -> w547
                        tunnel: w544 -> [w549 _]
                        tunnel: w545 -> [_ w550]
                        frame False {
                        }
                        frame True {
                        }
                      }
                      n194 = call "WaitMinTimeBetweenCall.vi"("Minimum ms between calls"=w547) -> ()  [unwired: 2 in]
                    }
                    frame Default {
                      n195 = To Single Precision Float(number=w567) -> (single precision float=w554:sgl[])
                      n196 = Decimate 1D Array(w554) -> (w560:sgl[], w563:sgl[], w562:sgl[], w561:sgl[], w559:sgl[], w558:sgl[], w557:sgl[], w556:sgl[], w555:sgl[], w552:sgl[])
                      n197 = Build Array(w560, w563, w562, w561, w559, w558, w557, w556, w555, w552) -> (w553:sgl[][])
                      n198 = for {
                        tunnel: T6."little-endian" ("byte order (0:big-endian, network order)") -> [w577]
                        shift-right: [w571] -> w568
                        shift-left: w566 -> [w572]
                        tunnel: w553 -> [w575] mode=indexing
                        tunnel: w565 -> [w574] mode=indexing
                        tunnel: [w573] -> w564 mode=indexing
                        n199 = Write to Binary File(file (use dialog)=w574, data=w575, error in=w572, 5:FALSE ("prepend array or string size? (T)"), 9:w577) -> (refnum out=w573:refnum<file>, error out=w571:errorcluster)  [unwired: 2 out]
                      }
                    }
                  }
                  n200 = xnode "Read/Write Control"("FPGA VI Reference In"=w493, "error in"=w498) -> ("FPGA VI Reference Out"=w511:refnum<k20>, "error out"=w510:errorcluster, "Parar"=w489:bool, "Nº Ruedas 1"=→"Nº Ruedas 1":i32, "NºRuedas 2"=→"NºRuedas 2":i32)
                  "Parar" <- w489
                  n201 = case shown="False" w489 {
                    tunnel: [w527 w535] -> w490
                    tunnel: [w528 0.0] -> w504
                    frame False {
                      n202 = local read "Inicio pasada"() -> (w531:timestamp)
                      n203 = local read "Tiempo de adquisicion"() -> (w523:dbl)
                      n204 = Get Date/Time In Seconds() -> (seconds since 1Jan1904=w530:timestamp)
                      n205 = To Double Precision Float(number=w530) -> (double precision float=w529:dbl)
                      n206 = To Double Precision Float(number=w531) -> (double precision float=w532:dbl)
                      n207 = Subtract(x=w529, y=w532) -> (x-y=w528:dbl)
                      "Tiempo de paso (s)" <- w528
                      n208 = local write "Tiempo"(w529) -> ()
                      n209 = local read "Boton Adquirir?"() -> (w524:bool)
                      n210 = Greater?(x=w528, y=w523) -> (0:w526:bool)
                      n211 = Select(t=w526, s=w524, f=FALSE) -> (s? t:f=w527:bool)
                    }
                    frame True {
                      n212 = local read "Tiempo"() -> (w539:dbl)
                      n213 = local read "Tiempo extra al detector de paso (s)"() -> (w534:dbl)
                      n214 = Get Date/Time In Seconds() -> (seconds since 1Jan1904=w536:timestamp)
                      n215 = To Double Precision Float(number=w536) -> (double precision float=w537:dbl)
                      n216 = Subtract(x=w537, y=w539) -> (x-y=w538:dbl)
                      n217 = Greater?(x=w538, y=w534) -> (0:w535:bool)
                    }
                  }
                  "Fin" <- w490
                  n218 = local read "Timeout ruedas"() -> (w488:dbl)
                  n219 = xnode ("CheckLate")("FPGA VI Reference In"=w511, "error in"=w510) -> ("FPGA VI Reference Out"=w495:refnum<k20>, "error out"=w506:errorcluster, "Buffer Underflow"=→"Buffer Underflow":bool, "Buffer Overflow"=w497:bool)
                  "Buffer Overflow" <- w497
                  n220 = Greater?(x=w504, y=w488) -> (0:w502:bool)
                  "Timeout ruedas" <- w502
                  n221 = call "ErrorOverFlow.vi"("Buffer Overflow"=w497) -> ("error out"=w505:errorcluster)
                  n222 = Merge Errors(w506, w505) -> (w494:errorcluster)
                  n223 = Unbundle By Name(w499) -> ("status"=w503:bool)
                  n224 = Unbundle By Name(w494) -> ("status"=w508:bool)
                  n225 = Compound Arithmetic op=OR(w508, w490, w502, w503) -> (w518:bool)
                  "result" <- w518
                  n226 = case "Flush" shown="True" w518 {
                    tunnel: [w578 w583] -> w522
                    tunnel: [w579 w582] -> w517
                    tunnel: w495 -> [w579 w581]
                    tunnel: w494 -> [w578 w580]
                    frame False {
                    }
                    frame True {
                      n227 = xnode "Invoke Method"("FPGA VI Reference In"=w581, "error in"=w580) -> ("FPGA VI Reference Out"=w582:refnum<k20>, "error out"=w583:errorcluster)
                    }
                  }
                  "Block Size" <- w519
                  "Time to Acquire Block (ms)" <- w521
                }
                n228 = call <vilib>:"Watchdog Whack.vi"("error in (no error)"=w431, "reset watchdog after expire? (F)"=TRUE, "watchdogID in"=w432) -> ("error out"=w428:errorcluster, "watchdogID out"=w429:u64)  [unwired: 2 in, 1 out]
                n229 = local read "RFID LR6 on?"() -> (w427:bool)
                n230 = case shown="True" w427 {
                  tunnel: w434 -> [w446 w452]
                  tunnel: [w446 w451] -> w433
                  frame False {
                  }
                  frame True {
                    n231 = while {
                      shift-right: [w459] -> w451
                      shift-left: w452 -> [w460]
                      shift-right: [w458] -> w449
                      shift-left: string[] [] -> [w457]
                      shift-right: [w453] -> w447
                      shift-left: i32[] [] -> [w454]
                      i -> [w455]
                      stop <- w456 stop-if-true
                      n232 = case shown="No Error" w460 {
                        selector: w460 -> [w471 _]
                        tunnel: [w470 w486] -> w459
                        tunnel: [w466 string[] []] -> w458
                        tunnel: w457 -> [w465 _]
                        tunnel: w455 -> [w464 _]
                        tunnel: w454 -> [w463 _]
                        tunnel: [w462 i32[] []] -> w453
                        frame No Error {
                          n233 = call "LH6HD.vi"("error in (no error)"=w471, "Action"=enum16{"Init", "Start", "Read", "Stop", "Exit"}."Read") -> ("error out"=w470:errorcluster, "Tag"=w467:string)  [unwired: 8 in]
                          n234 = Not Equal?(x="", y=w467) -> (x != y?=w468:bool)
                          n235 = case shown="False" w468 {
                            tunnel: w467 -> [_ w480]
                            tunnel: [w474 w479] -> w466
                            tunnel: w465 -> [w474 w478]
                            tunnel: w464 -> [_ w475]
                            tunnel: w463 -> [w473 w477]
                            tunnel: [w473 w476] -> w462
                            frame False {
                            }
                            frame True {
                              n236 = Build Array (concatenate)(w478, w480) -> (w479:string[])
                              n237 = Build Array (concatenate)(w477, w475) -> (w476:i32[])
                            }
                          }
                        }
                        frame Error {
                          n238 = local read "LR6 IP address"() -> (w483:string)
                          n239 = local read "DeviceAddress"() -> (w481:u8)
                          n240 = local read "Port LR6"() -> (w484:u16)
                          n241 = call "LH6HD.vi"("DeviceAddress"=w481, "Reader Port"=w484, "IP Address"=w483, "Action"=enum16{"Init", "Start", "Read", "Stop", "Exit"}."Init") -> ("error out"=w486:errorcluster)  [unwired: 6 in, 1 out]
                        }
                      }
                      n242 = Wait Until Next ms Multiple(millisecond multiple=u32 500) -> ()  [unwired: 1 out]
                      n243 = local read "result"() -> (w456:bool)
                      "it-LR6" <- w455
                    }
                    "TAGs LR6" <- w449
                    "it-read-LR6" <- w447
                  }
                }
              }
              frame #2 {
                n244 = local read "RFID LR6 on?"() -> (w605:bool)
                n245 = Array Size(array=w623) -> (size(s)=w621:i32)
                n246 = local read "timeout ms (60000)"() -> (w608:i32)
                n247 = local read "AURA wheel test"() -> (w585:bool)
                n248 = case shown="True" w605 {
                  tunnel: w618 -> [w658 w664]
                  tunnel: [w658 w659] -> w617
                  frame False {
                  }
                  frame True {
                    n249 = call "LH6HD.vi"("error in (no error)"=w664, "Action"=enum16{"Init", "Start", "Read", "Stop", "Exit"}."Stop") -> ("error out"=w659:errorcluster)  [unwired: 8 in, 1 out]
                    n250 = call "Reporting_error.vi"("error out 2"=w659, "Concept"="Active RFID") -> ("Reporting"=w661:string)  [unwired: 1 in]
                    n251 = local read "Report"() -> (w662:string)
                    n252 = Concatenate Strings(w661, w662) -> (w660:string)
                    n253 = local write "Report"(w660) -> ()
                  }
                }
                n254 = local read "bytes to read"() -> (w607:i32)
                n255 = local read "RFID NEM on?"() -> (w606:bool)
                n256 = Decrement(x=w621) -> (x-1=w622:i32)
                n257 = local read "Puerto RFID"() -> (w638:u16)
                n258 = local read "RFID_Error"() -> (w648:errorcluster)
                n259 = local read "IP RFID"() -> (w620:string)
                n260 = local read "RFID_ID"() -> (w647:refnum<k5>)
                n261 = Index Array(array=w623, index=w622) -> (element=w631:refnum<file>)
                n262 = local write "result"(FALSE ("result")) -> ()
                n263 = xnode "Read/Write Control"("FPGA VI Reference In"=w604, "error in"=w603) -> ("FPGA VI Reference Out"=w649:refnum<k20>, "error out"=w600:errorcluster, "Chassis Temperature"=w657:i16)
                n264 = local read "TAGs LR6"() -> (w587:string[])
                n265 = case shown="True" w606 {
                  tunnel: w648 -> [w667 w680]
                  tunnel: w647 -> [w666 w679]
                  tunnel: [w666 w678] -> w646
                  tunnel: [w667 w668] -> w642
                  tunnel: w638 -> [_ w677]
                  tunnel: w620 -> [_ w676]
                  tunnel: [_ w675] -> w602
                  tunnel: w608 -> [_ w674]
                  tunnel: w607 -> [_ w673]
                  frame False {
                  }
                  frame True {
                    n266 = call "RFID_28_03_12.vi"("BYTES TO READ"=w673, "TIMEOUT"=w674, "RFID_Error"=w680, "Puerto RFID"=w677, "IP RFID"=w676, "RFID ID"=w679) -> ("RFID Error"=w668:errorcluster, "connection ID out"=w678:refnum<k5>, "TAGs HEX"=w675:string[])  [unwired: 1 in, 1 out]
                    n267 = call "Reporting_error.vi"("error out 2"=w668, "Concept"="Passive RFID") -> ("Reporting"=w670:string)  [unwired: 1 in]
                    n268 = local read "Report"() -> (w671:string)
                    n269 = Concatenate Strings(w670, w671) -> (w669:string)
                    n270 = local write "Report"(w669) -> ()
                  }
                }
                "TAGs HEX" <- w602
                n271 = Select(t=string[] ["A0000000000000000TESTNEM7", "A0000000000000000TESTNEM8"], s=w585, f=w587) -> (s? t:f=w584:string[])
                n272 = Divide(x=w657, y=4.0) -> (x/y=w596:dbl)
                "Temperatura (ºC)" <- w596
                n273 = local read "Tiempo de paso (s)"() -> (w644:dbl)
                n274 = for {
                  tunnel: w584 -> [w683] mode=indexing
                  tunnel: [w681] -> w611 mode=indexing
                  n275 = Search and Replace String(input string=w683, search string="00") -> (result string=w681:string)  [unwired: 6 in, 3 out]
                }
                n276 = local write "RFID_LR6_Error"(w617) -> ()
                n277 = Index Array(array=w602) -> (element=w616:string)  [unwired: 1 in]
                n278 = local read "Nº Ruedas 1"() -> (w594:i32)
                n279 = local read "NºRuedas 2"() -> (w598:i32)
                n280 = Not Equal?(x=w616, y="" ("delimiter (\\t)")) -> (x != y?=w614:bool)
                "Plataformas?" <- w614
                n281 = Multiply(x=w644, y=1000.0) -> (x*y=w595:dbl)
                n282 = case shown="True" w614 {
                  tunnel: w611 -> [w684 w685]
                  tunnel: [w684 w687] -> w597
                  tunnel: w602 -> [_ w686]
                  frame False {
                  }
                  frame True {
                    n283 = call "Union_TAGs_RFIDs.vi"("TAGs LR6"=w685, "TAGs HEX"=w686) -> ("TAGs"=w687:string[])
                  }
                }
                "TAGs" <- w597
                n284 = local write "RFID_ID"(w646) -> ()
                n285 = local write "RFID_Error"(w642) -> ()
                n286 = Build Array(w596, w595, w594, w598) -> (w599:dbl[])
                n287 = Build Array(w596, w595, w594) -> (w593:dbl[])
                n288 = local read "Direccion 0?"() -> (w592:bool)
                n289 = local read "Nombre de archivo"() -> (w630:path[])
                n290 = for {
                  shift-right: [w693] -> w636
                  shift-left: string[] [] -> [w692]
                  tunnel: w597 -> [w691] mode=indexing
                  n291 = Insert Into Array(array=w692, new element=w691) -> (w693:string[])  [unwired: 1 in]
                }
                n292 = Bundle("error out"=w600, w599, "TAGs"=w597, "Direccion 0?"=w592) -> (w591:T8)  [unwired: 1 in]
                n293 = Delete From Array(array=w630) -> (deleted portion=w629:path)  [unwired: 2 in, 1 out]
                n294 = To Single Precision Float(number=w593) -> (single precision float=w655:sgl[])
                n295 = xnode "Read/Write Control"("FPGA VI Reference In"=w649, "error in"=w600, "Stop"=TRUE ("stop")) -> ("FPGA VI Reference Out"=w633:refnum<k20>, "error out"=w632:errorcluster)
                n296 = call "Reporting_acqu.vi"("output cluster"=w591, "address repoting"=path "C:/Reporting/Reporting_adqu.txt" ("file (use dialog)")) -> ("Reporting"=w588:string)  [unwired: 1 in]
                n297 = Path To String(path=w629) -> (string=w635:string)
                n298 = local read "Report"() -> (w589:string)
                n299 = Write to Binary File(file (use dialog)=w631, data=w655, error in=w652, 5:FALSE ("prepend array or string size? (T)"), 9:T6."little-endian" ("byte order (0:big-endian, network order)")) -> (error out=w628:errorcluster)  [unwired: 3 out]
                n300 = local read "Timeout ruedas"() -> (w645:bool)
                n301 = Build Array (concatenate)(w635, w636) -> (w612:string[])
                n302 = local read "TAGS leidos"() -> (w624:path)
                n303 = Concatenate Strings(w588, w589) -> (w590:string)
                n304 = for {
                  shift-right: [w690] -> w639
                  shift-left: w628 -> [w689]
                  tunnel: w623 -> [w688] mode=indexing
                  n305 = Close File(refnum=w688, error in=w689) -> (error out=w690:errorcluster)  [unwired: 1 out]
                }
                n306 = local write "Report"(w590) -> ()
                n307 = xnode "Invoke Method"("FPGA VI Reference In"=w633, "error in"=w632) -> ("FPGA VI Reference Out"=w641:refnum<k20>, "error out"=w640:errorcluster)
                n308 = call-poly <vilib>:"Write Delimited Spreadsheet.vi"("file path (dialog if empty)"=w624, "1D data"=w612, "append to file? (F)"=TRUE ("transpose? (no:F)"), "transpose? (F)"=TRUE ("append to file? (new file:F)"), "delimiter (\\t)"=";" ("delimiter (\\t)")) -> ()  [unwired: 9 in, 2 out]
                n309 = Select(t="TEST", s=w645, f="Procesado") -> (s? t:f=w650:string)
              }
            }
            n310 = call <vilib>:"Watchdog Clear.vi"("error in (no error)"=w340, "watchdogID in"=w341) -> ("error out"=w342:errorcluster)  [unwired: 5 in]
            n311 = Unbundle By Name(w367) -> ("status"=w356:bool)
            n312 = Unbundle By Name(w365) -> ("status"=w357:bool)
            n313 = Merge Errors(w365, w342) -> (w364:errorcluster)
            n314 = Compound Arithmetic op=OR(w356, w357) -> (w354:bool)
            n315 = Select(t="TEST", s=w354, f=w355) -> (s? t:f=w352:string)
          }
          frame "Procesado" {
            n316 = flat-sequence {
              tunnel: w699 -> [w718]
              tunnel: [w718] -> w698
              tunnel: w697 -> [w714]
              tunnel: [w714] -> w696
              frame #0 {
                n317 = local read "Report"() -> (w715:string)
                n318 = call "Reporting_datetime.vi"() -> ("String"=w713:string)  [unwired: 11 in]
                n319 = Concatenate Strings(w713, "\nSTATUS: PROCESSING\nProcessing the measurement\n\n", w715) -> (w717:string)
                n320 = local write "Report"(w717) -> ()
              }
            }
            n321 = local read "Watchdog config"() -> (w705:T1)
            n322 = call <vilib>:"Watchdog Configure.vi"("error in (no error)"=w708, "expiration actions"=w705, "timeout (1 sec)"=300.0) -> ("error out"=w707:errorcluster, "watchdogID"=w704:u64)  [unwired: 1 in, 2 out]
            n323 = flat-sequence {
              tunnel: w707 -> [w725]
              tunnel: w704 -> [w721]
              tunnel: [w720] -> w703
              tunnel: [w719] -> w702
              tunnel: [w936] -> w701
              tunnel: w703 -> [w936]
              tunnel: [w935] -> w700
              tunnel: w702 -> [w935]
              frame #0 {
                n324 = flat-sequence {
                  tunnel: [w797] -> w727
                  tunnel: [w783] -> w726
                  tunnel: w725 -> [w764]
                  tunnel: [w746] -> w722
                  tunnel: [w785] -> w724
                  tunnel: [w737] -> w723
                  tunnel: w721 -> [w765]
                  tunnel: [w762] -> w720
                  tunnel: [w761] -> w719
                  frame #0 {
                    n325 = local read "AURA wheel test"() -> (w735:bool)
                    n326 = case shown="True" w735 {
                      tunnel: [w800 w801] -> w734
                      tunnel: [w799 path[] [path "c:/Trenes_prueba/A_0_TEST.bin", path "c:/Trenes_prueba/A_1_TEST.bin", path "c:/Trenes_prueba/A_2_TEST.bin", path "c:/Trenes_prueba/A_3_TEST.bin", path "c:/Trenes_prueba/A_4_TEST.bin", path "c:/Trenes_prueba/A_5_TEST.bin", path "c:/Trenes_prueba/A_6_TEST.bin", path "c:/Trenes_prueba/A_7_TEST.bin", path "c:/Trenes_prueba/I_0_TEST.bin", path "c:/Trenes_prueba/I_1_TEST.bin"]] -> w733
                      frame False {
                        n327 = local read "Nombre de archivo"() -> (w799:path[])
                        n328 = local read "TAGs"() -> (w800:string[])
                      }
                      frame True {
                        w801 = string[] ["A0000000000000000TESTNEM7", "A0000000000000000TESTNEM8"]
                        n329 = local write "TAGs LR6"(w801) -> ()
                      }
                    }
                    n330 = local read "Tabla_flota"() -> (w782:string[][])
                    n331 = call <vilib>:"Watchdog Whack.vi"("error in (no error)"=w764, "reset watchdog after expire? (F)"=TRUE, "watchdogID in"=w765) -> ("error out"=w761:errorcluster, "watchdogID out"=w762:u64)  [unwired: 2 in, 1 out]
                    n332 = local read "Puntos medios de las ventanas"() -> (w784:dbl[][])
                    n333 = call "Series_ejes_flota.vi"("Tabla_flota"=w782, "Tags"=w734) -> ("Nº Ejes"=w759:i32[], "Series del convoy"=w776:string[])  [unwired: 2 in, 1 out]
                    "Nº Ejes" <- w759
                    n334 = Array Size(array=w733) -> (size(s)=w791:i32)
                    n335 = Add Array Elements(numeric array=w759) -> (sum=w745:i32)
                    "Ejes_convoy" <- w745
                    n336 = Subtract(x=w791, y=2 ("length")) -> (x-y=w793:i32)
                    n337 = Array Size(array=w776) -> (size(s)=→"Nº UTs":i32)
                    n338 = local read "Series_flota"() -> (w781:string[])
                    n339 = Delete From Array(array=w733, length=2, index=w793) -> (deleted portion=w766:path[], array with subset deleted=w785:path[])
                    n340 = Index Array(array=w766) -> (element #2=w760:path)  [unwired: 2 in, 1 out]
                    n341 = call "Distancias_ejes_convoy.vi"("Series_flota1"=w776, "Ejes_UT"=w759, "Puntos medios de las ventanas"=w784, "Series_flota"=w781) -> ("Distancias_entre_ejes_convoy"=w783:dbl[])  [unwired: 1 in]
                    n342 = Read from Binary File(5:sgl 0.0, 9:T6."little-endian" ("byte order (0:big-endian, network order)"), 10:-1 ("count (1)"), 11:w760) -> (0:w789:errorcluster, 2:w768:sgl[], 3:w790:refnum<file>)  [unwired: 1 in, 2 out]
                    n343 = local read "Frecuencia de muestreo (Hz)"() -> (w750:dbl)
                    n344 = local read "Offset_rueda WS 2"() -> (w751:fxp<+/-,24,-4>)
                    n345 = local read "TAGs"() -> (w774:string[])
                    n346 = local read "it-LR6"() -> (w771:i32)
                    n347 = local read "it-read-LR6"() -> (w772:i32[])
                    n348 = local read "TAGs LR6"() -> (w773:string[])
                    n349 = local read "Plataformas?"() -> (w770:bool)
                    n350 = Close File(refnum=w790, error in=w789) -> (error out=w729:errorcluster)  [unwired: 1 out]
                    n351 = Array Size(array=w768) -> (size(s)=w780:i32)
                    n352 = Subtract(x=w780, y=3 ("length")) -> (x-y=w778:i32)
                    n353 = Delete From Array(array=w768, length=3, index=w778) -> (array with subset deleted=w757:sgl[])  [unwired: 1 out]
                    n354 = call "TAGs_AURAwheel.vi"("Nº Ejes"=w759, "TAGs"=w774, "Ejes_convoy"=w745, "it-LR6"=w771, "TAGs LR6"=w773, "it-read-LR6"=w772, "Plataformas?"=w770) -> ("TAGS_AURA"=→"TAGs_AURAwheel":string[][])  [unwired: 1 in]
                    n355 = call "Analogico_digital.vi"("Array"=w757, "Offset WS"=w751, "Frecuencia muestreo"=w750) -> ("array w/ subset deleted"=w752:sgl[], "Tiempo\npaso"=w749:dbl)  [unwired: 6 in]
                    n356 = call "Puntos medio de pulso.vi"("DI Inductivo"=w752) -> ("Puntos"=w797:sgl[], "Número de ejes"=w739:i32)  [unwired: 1 in]
                    "Número de ejes detectados" <- w739
                    n357 = disable-structure shown="Disabled" {
                      disable-tunnel: w757 -> [w809 w812]
                      disable-tunnel: [FALSE ("element") TRUE ("element")] -> w754
                      disable-tunnel: [w803 w811] -> w753
                      frame Disabled {
                        n358 = Equal?(x=w809, y=0.0) -> (x = y?=w806:bool[])
                        n359 = Equal?(x=w809, y=1.0) -> (x = y?=w807:bool[])
                        n360 = Or(x=w806, y=w807) -> (x .or. y?=w803:bool[])
                      }
                      frame Enabled {
                        n361 = Greater?(x=w812, y=0.1) -> (0:w811:bool[])
                      }
                    }
                    n362 = Decrement(x=w739) -> (x-1=w796:i32)
                    n363 = call "Reporting_error.vi"("error out 2"=w729, "Concept"="Measurement reading") -> ("Reporting"=w731:string)  [unwired: 1 in]
                    n364 = Get Volume Info(11:path "c:/" ("path")) -> (1:w740:i64)  [unwired: 1 in, 5 out]
                    "Disco Duro Disponible (bytes)" <- w740
                    n365 = local read "Report"() -> (w732:string)
                    n366 = call "Calculo_Velocidad.vi"("Tiempo de paso (s)"=w749, "Ejes"=w796, "Puntos iniciales de las ventanas"=w783) -> ("V (m/s)"=→"V (m/s)":dbl, "Longitud de la unidad"=→"Longitud de la unidad":dbl)
                    n367 = Concatenate Strings(w731, w732) -> (w730:string)
                    n368 = Equal?(x=w745, y=w739) -> (x = y?=w737:bool)
                    n369 = Not Equal?(x=w739, y=0) -> (x != y?=w736:bool)
                    n370 = Search 1D Array(1D array=w753, element=w754) -> (index of element=w755:i32)  [unwired: 1 in]
                    n371 = local write "Report"(w730) -> ()
                    n372 = Build Array(w745, w739, w740) -> (w744:i64[])
                    n373 = Equal?(x=w755, y=-1) -> (x = y?=w758:bool)
                    n374 = Compound Arithmetic op=AND(w737, w736, w758) -> (w746:bool)
                    "Archivo\nvalido?" <- w746
                    n375 = Bundle(w744, w746) -> (w742:cluster{i64[], bool})  [unwired: 1 in]
                    n376 = call "Reporting_proc.vi"("output cluster 2"=w742, "address repoting"=path "C:/Reporting/Reporting_proc.txt" ("file (use dialog)")) -> ("Reporting"=w741:string)  [unwired: 1 in]
                    n377 = local read "Report"() -> (w747:string)
                    n378 = Concatenate Strings(w741, w747) -> (w748:string)
                    n379 = local write "Report"(w748) -> ()
                  }
                }
                n380 = case shown="True" w722 {
                  tunnel: w727 -> [_ w847]
                  tunnel: w726 -> [_ w845]
                  tunnel: w724 -> [_ w846]
                  tunnel: w723 -> [w814 _]
                  frame False {
                    n381 = local read "Nombre de archivo"() -> (w815:path[])
                    n382 = for {
                      tunnel: w815 -> [w817] mode=indexing
                      tunnel: w814 -> [w816]
                      n383 = flat-sequence {
                        tunnel: w817 -> [w827]
                        tunnel: [w827] -> w820
                        tunnel: [w826] -> w819
                        tunnel: w816 -> [w825]
                        tunnel: w820 -> [w834]
                        tunnel: [w833] -> w818
                        tunnel: w819 -> [w833]
                        tunnel: w818 -> [w836]
                        frame #0 {
                          w826 = path "c:/Est_Adq.csv" ("file path (use dialog)")
                          n384 = Path To String(path=w827) -> (string=w828:string)
                          n385 = Select(t="Nº Ejes detectados WS diferente a Nº Ejes TAGs" ("delimiter (\\t)"), s=w825, f="La señal del inductivo no es digital" ("delimiter (\\t)")) -> (s? t:f=w822:string)
                          n386 = Build Array(w828, w822) -> (w821:string[])
                          n387 = call-poly <vilib>:"Write Delimited Spreadsheet.vi"("file path (dialog if empty)"=w826, "1D data"=w821, "append to file? (F)"=FALSE ("transpose? (no:F)"), "transpose? (F)"=TRUE ("append to file? (new file:F)"), "delimiter (\\t)"=";" ("delimiter (\\t)")) -> ()  [unwired: 9 in, 2 out]
                        }
                        frame #1 {
                          n388 = local read "Borrar archivos\nadquisicion con error"() -> (w832:bool)
                          n389 = case shown="True" w832 {
                            tunnel: w834 -> [_ w835]
                            frame False {
                            }
                            frame True {
                              n390 = Delete(path (use dialog)=w835) -> ()  [unwired: 1 in, 6 out]
                            }
                          }
                        }
                        frame #2 {
                          n391 = File/Directory Info(path=w836) -> (size=w839:i64)  [unwired: 1 in, 6 out]
                          n392 = Greater?(x=w839, y=i64 1000000) -> (0:w837:bool)
                          n393 = case shown="True" w837 {
                            tunnel: w836 -> [_ w840]
                            frame False {
                            }
                            frame True {
                              n394 = Delete(path (use dialog)=w840) -> ()  [unwired: 4 in, 3 out]
                            }
                          }
                        }
                      }
                    }
                  }
                  frame True {
                    n395 = flat-sequence {
                      tunnel: w847 -> [w924]
                      tunnel: w846 -> [w921]
                      tunnel: w845 -> [w925]
                      tunnel: [w908] -> w844
                      frame #0 {
                        # "SALIDA \n\nMáximos por rueda inductivo"
                        # "8 acelerómetros"
                        # "Velocidad"
                        n396 = local read "Frecuencia de muestreo (Hz)"() -> (w923:dbl)
                        n397 = local read "Distancia de acelerómetros"() -> (w913:dbl[])
                        n398 = local read "Parámetros acelerómetros"() -> (w920:dbl[])
                        n399 = local read "Número de ejes detectados"() -> (w919:i32)
                        n400 = local read "Distancias generales"() -> (w918:dbl[])
                        n401 = local read "dt RMS"() -> (w922:dbl)
                        n402 = local read "Direccion 0?"() -> (w910:bool)
                        n403 = Index Array(array=w918, index=1) -> (element=w916:dbl)
                        n404 = Select(t=0.0, s=w910, f=w916) -> (s? t:f=w914:dbl)
                        n405 = Subtract(x=w914, y=w913) -> (x-y=w912:dbl[])
                        n406 = Absolute Value(x=w912) -> (abs(x)=w911:dbl[])
                        n407 = call "Procesado_aRMS_BIdirecc.vi"("Paths_canales_aRMS"=w921, "Ejes Procesados"=w919, "Distancias\nacelerometros"=w911, "Distancias generales (m)"=w918, "Distancias centrales de las ruedas\n               configuración (m)"=w925, "Frecuencia de muestreo"=w923, "Parámetros acelerómetros"=w920, "dt RMS 2"=w922, "Puntos"=w924) -> ("Max RMS Ruedas"=w909:dbl[][])  [unwired: 2 in]
                        n408 = Transpose 2D Array(2D array=w909) -> (transposed array=w908:dbl[][])
                        "Max RMS Ruedas" <- w908
                        n409 = call "Reporting_proc_RMS.vi"("Max RMS Ruedas"=w908) -> ("String"=w906:string)
                        n410 = local read "Report"() -> (w907:string)
                        n411 = Concatenate Strings(w906, w907) -> (w905:string)
                        n412 = local write "Report"(w905) -> ()
                      }
                    }
                    n413 = local read "Use Aura?"() -> (w843:bool)
                    n414 = local read "TAGs_AURAwheel"() -> (w842:string[][])
                    n415 = local read "Nº Ejes"() -> (w841:i32[])
                    n416 = for {
                      tunnel: w843 -> [w851]
                      tunnel: w842 -> [w850] mode=indexing
                      shift-right: [w849] -> _
                      shift-left: w844 -> [w852]
                      tunnel: w841 -> [w848] mode=indexing
                      # "dev.api.aurawheel.com"
                      n417 = case shown="True" w851 {
                        tunnel: w852 -> [w853 w872]
                        tunnel: w850 -> [_ w873]
                        tunnel: [w853 w871] -> w849
                        tunnel: w848 -> [_ w869]
                        frame False {
                        }
                        frame True {
                          w857 = "\n"
                          w880 = cluster{"status":string} {"status"=""}
                          n418 = local read "Parametros AuraWheel"() -> (w904:string[])
                          n419 = Delete From Array(array=w872, length=w869, index (row)=0) -> (deleted portion=w868:dbl[][], array with subset deleted=w871:dbl[][])  [unwired: 1 in]
                          n420 = Get Date/Time In Seconds() -> (seconds since 1Jan1904=w901:timestamp)
                          n421 = Format Date/Time String(time format string (%c)="%H:%M:%S%3u", seconds (now)=w901) -> (date/time string=w899:string)  [unwired: 1 in]
                          n422 = Get Date/Time In Seconds() -> (seconds since 1Jan1904=w876:timestamp)
                          n423 = Scan From String(format string="%d:%d:%f", input string=w899) -> (output 1=w896:i32, output 2=w895:i32, output 3=w893:dbl)  [unwired: 5 in, 3 out]
                          n424 = local read "V (m/s)"() -> (w864:dbl)
                          n425 = local read "Temperatura (ºC)"() -> (w874:dbl)
                          n426 = Multiply(x=w864, y=3.6) -> (x*y=w862:dbl)
                          n427 = Multiply(x=w893, y=1000.0) -> (x*y=w889:dbl)
                          n428 = call "Time_to_ms.vi"("seconds since 1Jan1904"=w876) -> ("Numeric"=w875:dbl)  [unwired: 1 in]
                          n429 = Multiply(x=w895, y=60000) -> (x*y=w890:i32)
                          n430 = Multiply(x=3600000, y=w896) -> (x*y=w891:i32)
                          n431 = Index Array(array=w904) -> (element #1=w867:string, element #2=w866:string, element #3=w865:string)  [unwired: 3 in]
                          n432 = call "aw_WRDCluster_8acel.vi"("Array TAGs"=w873, "Max RMS Ruedas"=w868, "TimeStamp"=w875, "p_sp"=w862, "p_tp"=w874) -> ("JSON cluster"=w902:T9)  [unwired: 1 in]
                          n433 = Compound Arithmetic op=ADD(w891, w890, w889) -> (w888:dbl)
                          n434 = To Variant(anything=w902) -> (Variant=w885:variant)
                          n435 = To Unsigned Long Integer(number=w888) -> (unsigned 32bit integer=w887:u32)
                          n436 = call "gjson_Create.vi"("JSON Object in"=w885) -> ("error out"=w883:errorcluster, "JSON String Out"=w884:string)  [unwired: 9 in]
                          n437 = Number To Decimal String(number=w887) -> (decimal integer string=w886:string)  [unwired: 1 in]
                          n438 = To Variant(anything=w880) -> (Variant=w879:variant)
                          n439 = call "aw_SendData.vi"("pwd"=w867, "x-nem-datetime"=w886, "User"=w866, "error in"=w883, "JSON Object"=w884, "URL"=w865) -> ("error out"=w881:errorcluster, "Response JSON"=w882:string, "Response headers"=w858:string)  [unwired: 3 in]
                          "Response headers" <- w858
                          n440 = call "gjson_Parse.vi"("error in"=w881, "JSON String In"=w882, "JSON Cluster"=w879) -> ("error out"=w877:errorcluster, "JSON Cluster Out"=w878:variant)  [unwired: 7 in]
                          n441 = Variant To Data(error in=w877, type=w880, Variant=w878) -> (data=→"data":cluster{"status":string}, error out=w859:errorcluster)
                          "error AURA" <- w859
                          n442 = local read "Report"() -> (w855:string)
                          n443 = call "Reporting_error.vi"("error out 2"=w859, "Concept"="A.U.R.A. Wheel Connection") -> ("Reporting"=w860:string)  [unwired: 1 in]
                          n444 = Concatenate Strings(w860, w857, w857, w858, w857) -> (w856:string)
                          "Report_AURA" <- w856
                          n445 = Concatenate Strings(w856, w855) -> (w854:string)
                          n446 = local write "Report"(w854) -> ()
                        }
                      }
                    }
                  }
                }
              }
              frame #1 {
                n447 = local read "Archivo\nvalido?"() -> (w932:bool)
                n448 = local read "Bytes libre despues de borrar"() -> (w933:u32)
                n449 = local read "Report_AURA"() -> (w929:string)
                n450 = local read "Max archivos"() -> (w930:u32)
                n451 = local read "Path LOG"() -> (w931:path)
                n452 = local read "LOG.txt"() -> (w926:path)
                n453 = local read "Report"() -> (w928:string)
                n454 = local read "Bytes min libre"() -> (w934:u32)
                n455 = local read "TAGS leidos"() -> (w937:path)
                n456 = File/Directory Info(path=w937) -> (size=w940:i64)  [unwired: 1 in, 6 out]
                n457 = case shown="True" w932 {
                  frame False {
                  }
                  frame True {
                    n458 = local read "Nombre de archivo"() -> (w942:path[])
                    n459 = call "Comprimir_a_1_archivo.vi"("Acel_paths"=w942) -> ("path_Pasada"=→"created path":path)
                  }
                }
                n460 = Greater?(x=w940, y=i64 1000000) -> (0:w938:bool)
                n461 = case shown="True" w938 {
                  tunnel: w937 -> [_ w943]
                  frame False {
                  }
                  frame True {
                    n462 = Delete(path (use dialog)=w943) -> ()  [unwired: 4 in, 3 out]
                  }
                }
                n463 = call "BORRADO_MEJORADO_Gonzalo.vi"("Bytes LIBRE OK"=w933, "Bytes Minimo de Memoria libre"=w934) -> ()  [unwired: 10 in]
                n464 = call "Saving_LOG.vi"("Path"=w926, "Report"=w928, "Report AURA"=w929, "Path Carpeta"=w931, "Nº Archivos Max"=w930) -> ("Report"=w927:string)  [unwired: 9 in, 1 out]
                n465 = local write "Report"(w927) -> ()
              }
            }
            n466 = call <vilib>:"Watchdog Clear.vi"("error in (no error)"=w700, "watchdogID in"=w701) -> ("error out"=w694:errorcluster)  [unwired: 5 in]
            n467 = Merge Errors(w696, w694) -> (w712:errorcluster)
            n468 = Unbundle By Name(w712) -> ("status"=w710:bool)
            n469 = Select(t="TEST", s=w710, f="Espera") -> (s? t:f=w709:string)
          }
          frame "TEST" {
            n470 = flat-sequence {
              tunnel: w948 -> [w959]
              tunnel: [w959] -> w946
              frame #0 {
                n471 = call "Reporting_datetime.vi"() -> ("String"=w958:string)  [unwired: 11 in]
                n472 = local read "Report"() -> (w960:string)
                n473 = Concatenate Strings(w958, "\nSTATUS: ERROR TEST\n\n", w960) -> (w962:string)
                n474 = local write "Report"(w962) -> ()
              }
            }
            n475 = local read "Watchdog config"() -> (w953:T1)
            n476 = call <vilib>:"Watchdog Configure.vi"("error in (no error)"=w944, "expiration actions"=w953, "timeout (1 sec)"=200.0) -> ("error out"=w954:errorcluster, "watchdogID"=w951:u64)  [unwired: 1 in, 2 out]
            n477 = Merge Errors(w946, w944) -> (w945:errorcluster)
            n478 = flat-sequence {
              tunnel: [w972] -> w957
              tunnel: w954 -> [w967]
              tunnel: w945 -> [w985]
              tunnel: [w968] -> w955
              tunnel: w951 -> [w966]
              tunnel: [w965] -> w950
              tunnel: [w964] -> w949
              frame #0 {
                n479 = call <vilib>:"Watchdog Whack.vi"("error in (no error)"=w967, "reset watchdog after expire? (F)"=TRUE, "watchdogID in"=w966) -> ("error out"=w964:errorcluster, "watchdogID out"=w965:u64)  [unwired: 2 in, 1 out]
                n480 = Get Date/Time In Seconds() -> (seconds since 1Jan1904=w979:timestamp)
                n481 = local read "Ultimo TEST"() -> (w980:timestamp)
                n482 = To Double Precision Float(number=w979) -> (double precision float=w981:dbl)
                n483 = Subtract(x=w981, y=3600.0) -> (x-y=w983:dbl)
                n484 = To Time Stamp(1:w983) -> (0:w984:timestamp)
                n485 = In Range and Coerce(upper limit=w979, x=w980, lower limit=w984) -> (In Range?=w978:bool)  [unwired: 1 out]
                n486 = case shown="False" w978 {
                  tunnel: w985 -> [w995 w1019]
                  tunnel: [w995 w1019] -> w968
                  frame False {
                    n487 = local read "Timeout ruedas"() -> (w996:bool)
                    n488 = local read "Aviso no detección"() -> (w999:string)
                    n489 = local read "Aviso temperatura"() -> (w998:string)
                    n490 = case shown="True" w996 {
                      selector: w996 -> [_ w1016]
                      tunnel: ["\r" w1017] -> w994
                      frame False {
                      }
                      frame True {
                        w1006 = "\n"
                        n491 = local read "Nº Ruedas 1"() -> (w1013:i32)
                        n492 = local read "NºRuedas 2"() -> (w1008:i32)
                        n493 = call "ErrorRuedas.vi"("Buffer Overflow"=w1016) -> ("error out"=w1018:errorcluster)
                        n494 = Number To Decimal String(number=w1013) -> (decimal integer string=w1011:string)  [unwired: 1 in]
                        n495 = Number To Decimal String(number=w1008) -> (decimal integer string=w1007:string)  [unwired: 1 in]
                        n496 = Concatenate Strings("Error Wheel sensors", "\n", "WS1 (wheels):", w1011, w1006, "WS2 (wheels):", w1007, w1006) -> (w1009:string)
                        n497 = call "Error.vi"("Error con..."=w1009, "error comunicacion 2"=w1018) -> ("String"=w1017:string)
                      }
                    }
                    n498 = local read "DC OK"() -> (w997:string)
                    n499 = call "Cabecera.vi"() -> ("String"=w1004:string)
                    n500 = call "Adquisicion.vi"("Aviso no detección"=w999) -> ("String"=w1003:string)
                    n501 = call "Temperatura.vi"("Aviso temperatura"=w998) -> ("String"=w1002:string)
                    n502 = call "Fuente.vi"("DC OK"=w997) -> ("String"=w1001:string)
                    n503 = call "FPGA.vi"("error out"=w995) -> ("String"=w1000:string)
                    n504 = Concatenate Strings(w1004, w1003, w1002, w1001, w1000, w994) -> (w987:string)
                    n505 = local read "Report"() -> (w986:string)
                    n506 = Get Date/Time In Seconds() -> ()  [unwired: 1 out]
                    n507 = Concatenate Strings(w987, w986) -> (w989:string)
                    n508 = local read "Max archivos"() -> (w990:u32)
                    n509 = local read "Path LOG"() -> (w993:path)
                    n510 = local read "LOG.txt"() -> (w991:path)
                    n511 = call "Saving_LOG.vi"("Path"=w991, "Report"=w989, "Report AURA"=w987, "Path Carpeta"=w993, "Nº Archivos Max"=w990) -> ("Report"=w992:string)  [unwired: 9 in, 1 out]
                    n512 = local write "Report"(w992) -> ()
                    "Ultimo TEST" <- timestamp(3608692059.513 s since 1904-01-01) ("Ultimo TEST")
                  }
                  frame True {
                  }
                }
                n513 = local read "Fallo fotocelula"() -> (w971:bool)
                n514 = Unbundle By Name(w968) -> ("status"=w969:bool)
                n515 = local read "T fuera rango"() -> (w977:bool)
                n516 = Compound Arithmetic op=OR(w969, w971) -> (w970:bool)
                n517 = local write "Reset del controlador"(w970) -> ()
                n518 = Select(t="Escape", s=w977, f="Espera") -> (s? t:f=w974:string)
                n519 = Select(t="Configuracion", s=w970, f=w974) -> (s? t:f=w972:string)
              }
            }
            n520 = call <vilib>:"Watchdog Clear.vi"("error in (no error)"=w949, "watchdogID in"=w950) -> ("error out"=w947:errorcluster)  [unwired: 5 in]
          }
          frame "Calibracion" {
            n521 = flat-sequence {
              tunnel: w1035 -> [w1193]
              tunnel: w1034 -> [w1192]
              tunnel: [w1193] -> w1033
              tunnel: [w1192] -> w1032
              frame #0 {
                n522 = local read "Report"() -> (w1189:string)
                n523 = call "Reporting_datetime.vi"() -> ("String"=w1188:string)  [unwired: 11 in]
                n524 = Concatenate Strings(w1188, "\nSTATUS: CALIBRATION\n\n\n", w1189) -> (w1191:string)
                n525 = local write "Report"(w1191) -> ()
              }
            }
            n526 = flat-sequence {
              tunnel: w1032 -> [w1039]
              tunnel: w1033 -> [w1040]
              tunnel: [w1040] -> w1028
              tunnel: [w1039] -> w1027
              tunnel: [w1037] -> w1026
              tunnel: w1028 -> [w1045]
              tunnel: w1027 -> [w1044]
              tunnel: w1026 -> [w1041]
              tunnel: [w1043] -> w1025
              tunnel: [w1042] -> w1024
              tunnel: w1025 -> [w1156]
              tunnel: w1024 -> [w1155]
              tunnel: [w1156] -> w1023
              tunnel: [w1155] -> w1022
              tunnel: [w1137] -> w1021
              tunnel: [w1136] -> w1020
              tunnel: [w1174] -> w1029
              tunnel: [w1175] -> w1030
              tunnel: w1023 -> [w1175]
              tunnel: w1022 -> [w1174]
              tunnel: w1021 -> [w1173]
              tunnel: w1020 -> [w1169]
              frame #0 {
                n527 = call "Folder_creation_calibration.vi"() -> ("path"=w1038:path, "date/time string"=w1037:string, "calibration log"=→"calibration log":path)  [unwired: 2 in]
                "Folder" <- w1038
                n528 = Create Folder(path (use dialog)=w1038) -> ()  [unwired: 2 in, 3 out]
              }
              frame #1 {
                n529 = for {
                  N: 11 -> [_]
                  shift-right: [w1070] -> w1043
                  shift-left: w1045 -> [w1069]
                  shift-right: [w1071] -> w1042
                  shift-left: w1044 -> [w1068]
                  tunnel: w1041 -> [w1047]
                  i -> [w1063]
                  n530 = xnode "Invoke Method"("FPGA VI Reference In"=w1069, "error in"=w1068) -> ("FPGA VI Reference Out"=w1067:refnum<k20>, "error out"=w1065:errorcluster)  [unwired: 1 in]
                  n531 = Increment(x=w1063) -> (x+1=w1062:i32)
                  n532 = Number To Decimal String(number=w1062) -> (decimal integer string=w1061:string)  [unwired: 1 in]
                  n533 = flat-sequence {
                    tunnel: w1067 -> [w1135]
                    tunnel: [w1135] -> w1066
                    tunnel: w1065 -> [w1134]
                    tunnel: [w1134] -> w1064
                    tunnel: w1061 -> [w1133]
                    frame #0 {
                      n534 = local read "Report"() -> (w1130:string)
                      n535 = Concatenate Strings("\nAcquiring file: ", w1133, "/11\n" ("string"), w1130) -> (w1129:string)
                      n536 = local write "Report"(w1129) -> ()
                    }
                  }
                  n537 = flat-sequence {
                    tunnel: w1064 -> [w1074]
                    tunnel: w1066 -> [w1075]
                    tunnel: [w1075] -> w1060
                    tunnel: [w1074] -> w1059
                    tunnel: [w1072] -> w1048
                    tunnel: w1047 -> [w1072]
                    tunnel: [w1089] -> w1058
                    tunnel: [w1088] -> w1057
                    tunnel: [w1087] -> w1056
                    tunnel: [w1086] -> w1055
                    tunnel: [w1085] -> w1054
                    tunnel: [w1084] -> w1053
                    tunnel: w1060 -> [w1092]
                    tunnel: w1059 -> [w1091]
                    tunnel: w1048 -> [w1076]
                    tunnel: [w1115] -> w1052
                    tunnel: [w1100] -> w1051
                    tunnel: [w1114] -> w1050
                    tunnel: [w1099] -> w1049
                    tunnel: w1058 -> [w1113]
                    tunnel: w1057 -> [w1112]
                    tunnel: w1056 -> [w1111]
                    tunnel: w1055 -> [w1110]
                    tunnel: w1054 -> [w1109]
                    tunnel: w1053 -> [w1108]
                    tunnel: w1052 -> [w1125]
                    tunnel: w1051 -> [w1124]
                    tunnel: w1050 -> [w1126]
                    tunnel: w1049 -> [w1116]
                    tunnel: [w1127] -> w1071
                    tunnel: [w1128] -> w1070
                    frame #0 {
                      n538 = Wait (ms)(milliseconds to wait=u32 1000) -> ()  [unwired: 1 out]
                    }
                    frame #1 {
                      n539 = local read "Frecuencia de muestreo y módulo CRIO"() -> (w1093:T2)
                      n540 = local read "Escaneos de la FIFO por canal"() -> (w1096:u32)
                      n541 = local read "Frecuencia de muestreo (Hz)"() -> (w1095:dbl)
                      n542 = local read "Nº de acelerómetros"() -> (w1098:i32)
                      n543 = local read "Nº inductivos"() -> (w1097:i32)
                      n544 = local read "Count(mSec)"() -> (w1094:u32)
                      n545 = Get Date/Time In Seconds() -> (seconds since 1Jan1904=→"Inicio pasada 2":timestamp)
                      n546 = Bundle("Frecuencia de muestreo y módulo CRIO"=w1093, "Count(mSec)"=w1094, "Frecuencia de muestreo (Hz)"=w1095, "Escaneos de la FIFO por canal"=w1096, "Nº inductivos"=w1097, "Nº de acelerómetros"=w1098) -> (w1090:T10)  [unwired: 1 in]
                      n547 = call "Config_calibr.vi"("error in (no error)"=w1091, "Date Folder"=w1076, "Acq parameters"=w1090, "Refnum in"=w1092) -> ("error out"=w1088:errorcluster, "Block Size"=w1086:u32, "Time to Acquire Block (ms)"=w1087:i32, "Refnum out"=w1089:refnum<k20>, "refnum out"=w1085:refnum<file>, "path"=w1078:path, "error out 2"=w1084:errorcluster)  [unwired: 1 in]
                      "path calib" <- w1078
                      n548 = Path To String(path=w1078) -> (string=w1079:string)
                      n549 = local read "Report"() -> (w1083:string)
                      n550 = Concatenate Strings("\nFile created: ", w1079, "\n", w1083) -> (w1082:string)
                      n551 = local write "Report"(w1082) -> ()
                    }
                    frame #2 {
                      n552 = local read "Inicio pasada 2"() -> (w1107:timestamp)
                      n553 = call "Acq_calibr.vi"("Refnum in"=w1113, "refnum in"=w1109, "Time to Acquire Block (ms)"=w1111, "Block Size"=w1110, "error out 3"=w1108, "error in (no error)"=w1112, "Inicio pasada 3"=w1107) -> ("refnum out 2"=w1114:refnum<file>, "Refnum out"=w1115:refnum<k20>, "Buffer Underflow 2"=w1106:bool, "error out 4"=w1100:errorcluster, "Buffer Overflow 2"=w1105:bool, "error out"=w1099:errorcluster)  [unwired: 3 in]
                      n554 = local write "Buffer Overflow"(w1105) -> ()
                      n555 = call "Reporting_error.vi"("error out 2"=w1100, "Concept"="FPGA ") -> ("Reporting"=w1102:string)  [unwired: 1 in]
                      n556 = local read "Report"() -> (w1103:string)
                      n557 = local write "Buffer Underflow"(w1106) -> ()
                      n558 = Concatenate Strings(w1102, w1103) -> (w1101:string)
                      n559 = local write "Report"(w1101) -> ()
                    }
                    frame #3 {
                      n560 = xnode "Read/Write Control"("FPGA VI Reference In"=w1125, "error in"=w1124, "Stop"=TRUE ("stop")) -> ("FPGA VI Reference Out"=w1123:refnum<k20>, "error out"=w1122:errorcluster)
                      n561 = call "Reporting_error.vi"("error out 2"=w1116, "Concept"="Saving file ") -> ("Reporting"=w1119:string)  [unwired: 1 in]
                      n562 = Close File(refnum=w1126, error in=w1116) -> ()  [unwired: 2 out]
                      n563 = local read "Report"() -> (w1118:string)
                      n564 = xnode "Invoke Method"("FPGA VI Reference In"=w1123, "error in"=w1122) -> ("FPGA VI Reference Out"=w1128:refnum<k20>, "error out"=w1127:errorcluster)
                      n565 = Concatenate Strings(w1119, w1118) -> (w1120:string)
                      n566 = local write "Report"(w1120) -> ()
                    }
                  }
                }
              }
              frame #2 {
                n567 = local read "Frecuencia de muestreo (Hz)"() -> (w1150:dbl)
                n568 = local read "Nº de acelerómetros"() -> (w1140:i32)
                n569 = local read "Nº inductivos"() -> (w1139:i32)
                n570 = local read "Pattern amplitude (g)"() -> (w1141:dbl)
                n571 = local read "Pattern frequency (Hz)"() -> (w1142:dbl)
                n572 = local read "Folder"() -> (w1154:path)
                n573 = Add(x=w1140, y=w1139) -> (x+y=w1138:i32)
                n574 = call <vilib>:"Recursive File List.vi"("Folder Path"=w1154) -> ("All Files in Dir"=w1153:path[])  [unwired: 6 in, 4 out]
                n575 = flat-sequence {
                  tunnel: w1148 -> [w1157]
                  tunnel: w1145 -> [w1160]
                  tunnel: w1144 -> [w1163]
                  tunnel: w1143 -> [w1166]
                  frame #0 {
                    n576 = local read "Report"() -> (w1158:string)
                    n577 = Concatenate Strings(w1157, w1158) -> (w1159:string)
                    n578 = local write "Report"(w1159) -> ()
                  }
                  frame #1 {
                    n579 = local read "Report"() -> (w1161:string)
                    n580 = Concatenate Strings(w1160, w1161) -> (w1162:string)
                    n581 = local write "Report"(w1162) -> ()
                  }
                  frame #2 {
                    n582 = local read "Report"() -> (w1165:string)
                    n583 = Concatenate Strings(w1163, w1165) -> (w1164:string)
                    n584 = local write "Report"(w1164) -> ()
                  }
                  frame #3 {
                    n585 = local read "Report"() -> (w1167:string)
                    n586 = Concatenate Strings(w1166, w1167) -> (w1168:string)
                    n587 = local write "Report"(w1168) -> ()
                  }
                }
                n588 = call "Acel_calib_detector.vi"("Frecuencia\nmuestreo"=w1150, "Pattern frequency (Hz)"=w1142, "Nº canales"=w1138, "All Files in Dir"=w1153) -> ("Reporting"=w1148:string, "Acceler.\ndetected"=w1137:i32, "Acel Cal measurements"=w1152:sgl[][])  [unwired: 1 out]
                n589 = call "Acel_calib_frequency.vi"("Pattern frequency (Hz)"=w1142, "Frecuencia\nmuestreo"=w1150, "Acel Cal measurements in"=w1152) -> ("Reporting2"=w1145:string, "Acel Cal measurements out"=w1151:sgl[][])  [unwired: 1 in, 2 out]
                n590 = call "Acel_calib_noise_files_out.vi"("Pattern frequency (Hz)"=w1142, "Frecuencia\nmuestreo"=w1150, "Acel Cal measurements in"=w1151) -> ("Reporting 3"=w1144:string, "Acel Cal measurements out 2"=w1149:sgl[][])  [unwired: 6 in, 1 out]
                n591 = call "Acel_calib_calib.vi"("Acel Cal measurements in"=w1149, "Frecuencia\nmuestreo"=w1150, "Pattern frequency (Hz)"=w1142, "Pattern\namplitude"=w1141) -> ("Calibration parameter"=w1136:dbl, "Reporting 4"=w1143:string)  [unwired: 7 in, 3 out]
                n592 = local read "calibration log"() -> (w1146:path)
                n593 = Concatenate Strings(w1148, w1145, w1144, w1143) -> (w1147:string)
                n594 = Write to Text File(file (use dialog)=w1146, text=w1147) -> ()  [unwired: 2 in, 3 out]
              }
              frame #3 {
                n595 = local read "Save calibration"() -> (w1170:bool)
                n596 = Add(x=w1173, y=8) -> (x+y=w1171:i32)
                n597 = case shown="True" w1170 {
                  tunnel: w1171 -> [_ w1185]
                  tunnel: w1169 -> [_ w1178]
                  frame False {
                  }
                  frame True {
                    w1186 = "Parametros"  # Key 1
                    n598 = local read "configuration file path"() -> (w1179:path)
                    n599 = Number To Decimal String(number=w1185) -> (decimal integer string=w1187:string)  [unwired: 1 in]
                    n600 = Concatenate Strings(w1186, w1187) -> (w1177:string)
                    n601 = call <vilib>:"Open Config Data.vi"("create file if necessary (T)"=TRUE, "configuration file path"=w1179) -> ("error out"=w1180:errorcluster, "refnum"=w1181:T11)  [unwired: 1 in, 7 out]
                    n602 = call-poly <vilib>:"Write Key.vi"("section"="Adquisicion", "error in (no error)"=w1180, "value"=w1178, "key"=w1177, "refnum"=w1181) -> ("error out"=w1184:errorcluster, "refnum out"=w1183:T11)  [unwired: 3 in, 2 out]
                    n603 = call <vilib>:"Close Config Data.vi"("error in (no error)"=w1184, "refnum"=w1183) -> ()  [unwired: 8 in, 2 out]
                  }
                }
              }
            }
          }
        }
        "error manipulacion archivos" <- w96
        n604 = local read "Parar la aplicación"() -> (w94:bool)
      }
      n605 = xnode "Close FPGA VI Reference"("FPGA VI Reference In"=w86, "error in"=w85) -> ("error out"=→"error FPGA":errorcluster)
    }
    frame #3 {
      n606 = local read "RFID_ID"() -> (w1196:refnum<k5>)
      n607 = call "LH6HD.vi"("Action"=enum16{"Init", "Start", "Read", "Stop", "Exit"}."Stop") -> ("error out"=→"RFID_LR6_Error":errorcluster)  [unwired: 9 in, 1 out]
      n608 = TCP Close Connection(connection ID=w1196) -> (error out=→"RFID_Error":errorcluster)  [unwired: 1 in, 2 out]
    }
  }
